vi "Main.vi"() -> ()   [LabVIEW 2015]
uses:
  Ctrls/btnCloseWin.ctl
  Ctrls/YesOrNo.ctl
  Ctrls/btnAboutNew.ctl
  Ctrls/btnDonateNew.ctl
  Ctrls/btnMinSizeWin.ctl
  Ctrls/btnMaxSizeWin.ctl
  Ctrls/btnUpdateNew.ctl
  Ctrls/btnOpenDBplusplus.ctl
  Ctrls/btnOpenCANtest.ctl
  Ctrls/btnOpenCANpro.ctl
  Ctrls/btnOpenZCANPRO.ctl
  Ctrls/btnSetupNew.ctl
  Ctrls/SettingParameters.ctl
  Ctrls/btnOpenDBC.ctl
  Ctrls/btnOpenData.ctl
  Ctrls/btnOpenTSmaster.ctl
  Ctrls/btnOpenOrigin.ctl
  <vilib>/Utility/sysdir.llb/System Directory Type.ctl
  <vilib>/Platform/TimedLoop/XDataNode/timing_clust.ctl
  <vilib>/Platform/TimedLoop/XDataNode/nitl_modes.ctl
  <vilib>/Platform/TimedLoop/XDataNode/wakeup.ctl
  <vilib>/Utility/miscctls.llb/LVPointTypeDef.ctl
  <vilib>/Utility/miscctls.llb/LVRectTypeDef.ctl
  SubVIs/GlobalVar.vi
  GlobalVariables.vi
  <vilib>/Utility/config.llb/Write Key (Boolean).vi
  <vilib>/Utility/config.llb/Read Key (Path).vi
  <vilib>/Utility/config.llb/Write Key (Path).vi
  <vilib>/Utility/config.llb/Read Key (Boolean).vi
  <vilib>/Utility/NIReport.llb/Append Text Table to Report (wrap).vi
  <vilib>/Platform/TimedLoop/XDataNode/XDataNode.xnode
  <vilib>/Utility/NIReport.llb/NI_report.lvclass
  <vilib>/Utility/config.llb/NI_LVConfig.lvlib
  <vilib>/Platform/TimedLoop/XDataNode/XDNodeRunTimeDep.lvlib
  <vilib>/Utility/NIReport.llb/Excel/NI_Excel.lvclass
panel:
  out "CursorNum2":dbl
  out "CursorNum1":dbl
  out "CursorTXT2":string
  out "CursorTXT1":string
  out "MainGrapgDraw_finished":bool
  out "Data_loaded":bool
  out "DBC_loaded":bool
  in  "btnMultiDecAndExp":bool caption="boolExport2Excel"
  in  "btnOpenOrigin":T1
  in  "btnOpenTSmaster":T2 caption="btnOpenCANpro"
  out "Y_DisplayNum":i32
  in  "ZoomMode":u16(ring) items=["Zoom：XY", "Zoom：X", "Zoom：Y1", "Zoom：Y2", "Zoom：Y3", "Zoom：Y4", "Zoom：Y5", "Zoom：Y6", "Zoom：Y7", "Zoom：Y8", "Zoom: All Y"]
  out "MporofSelSgs":string[][](array[string]) caption="已选信号数组"
  in  "btnOpenCANData":T3
  out "CANDatafileIn":string caption="CAN离线数据（.can/.txt/.csv/.asc/.trc/.blf）"
  in  "btnOpenDBC":T4
  out "DBCfileIn":string caption="DBC文件(.dbc)"
  in  "dbcSigOver1":bool
  in  "isShowYValue":T5=TRUE caption="AutoLine"
  in  "isShowXY":T5=TRUE caption="AutoLine"
  out "SelectedSigValListArry":string[][](array[string]) caption="值表数组"
  in  "LineWidth":u8
  out "XYTips":string
  out "ChkUpdateCnt":i32
  out "ReadSettingsReady":bool=TRUE
  out "Settings":T6 {"ChkUpdatePeriod" items=["EveryMonth"=2592000, "EveryWeek"=604800, "Everyday"=86400, "EveryHour"=3600, "EveryLaunch"=1, "Never"=0]}
  in  "btnConfigYandCurves":bool caption="配置纵坐标"
  in  "isAutoCurves":T5=TRUE caption="AutoLine"
  in  "isAutoY":T5=TRUE caption="AutoY"
  in  "TimeFormat":u16(ring) items=["Relative(s)", "Abs(noDate)", "Abs(withDate)"]
  in  "isTimeRerange":T5=TRUE caption="AutoY"
  out "Language":u32
  in  "btnSetup":T7
  in  "btnOpenZCANPRO":T8
  in  "btnOpenCANpro":T9
  in  "btnOpenCANtest":T10
  in  "btnOpenDBplus2":T11
  in  "btnUpdateChk":T12
  in  "btnMax":T13
  in  "btnMin":T14
  in  "btnCANFileInfo":bool caption="空白按钮"
  out "CANMessagesAllInfo":string[][](array[string])
  out "XYGraphData":cluster{"时间(s)":dbl[], "数据":dbl[]}[](array[cluster])
  out "BaseTimeCluster":T15
  in  "boolMergeFiles":bool caption="空白按钮"
  in  "btnDonate":T16
  in  "btnAbout":T17
  in  "ClusterSigFormat":T18
  out "CurveCustomSealedArray":string[][](array[string]) caption="已选信号数组"
  out "CanMessageRowsNum":i32 caption="帧数"
  out "FileSize":dbl caption="文件大小" format="%.2f MB"
  out "ManuCofigofYaxle":cluster{"Y轴序号":u8, "Y轴名称":string, "可见性":bool}[](array[cluster])
  out "ManuCofigofCurves":T19(array[cluster])
  in  "boolExport2Excel":bool
  out "LastCANPath":path
  out "LastDBCPath":path
  out "isDataLoaded":bool caption="离线数据已加载"
  out "DataArryOfCANLoaded":u32[][](array[numeric]) caption="加载的CAN离线数据数组"
  out "ProgressNumerical":string="0%" caption="进度数值"
  out "HorizontalProgressBar":u8(slide) caption="水平进度条" scale=0.0..100.0
  out "SigValListArry":string[][](array[string]) caption="值表数组"
  in  "LookAllSigDefinition":bool caption="查看所有值表"
  in  "LookSelSigDefinition":bool caption="查看已选值表"
  in  "AllValueTable":string(tree) caption="所有ValueTable"
  out "txtDrawingPrompt":string="让我看看有多少数据..." caption="绘图提示语"
  in  "GraphLegendWidth":u32 caption="图例与游标宽度"
  in  "ClearMainGraph":bool caption="清空主图"
  out "NumSelected":i32 caption="已选数量"
  in  "ListOfDBC":string(tree) caption="DBC一览树形"
  in  "boolLoadLastDBC":bool caption="空白按钮"
  in  "ClearSelectedSig":bool caption="清空选择"
  out "CANmessageNum":i32 caption="报文数"
  out "SigNum":i32 caption="信号数"
  in  "DBCpath":path caption="DBC文件（.dbc）"
  in  "CANpath":path caption="CAN离线数据（.can/.txt/.csv/.asc/.trc）"
  out "ArrySelectedSig":string[][](array[string]) caption="已选信号数组"
  out "DBCAllSigArry":string[][](array[string]) caption="全部信号数组"
  in  "boolDrawGraph":bool caption="绘图"
  in  "btnExit":T20 caption="退出"
  in  "SelectedSigList":i32(listbox)=-1 caption="已选信号列表"
  out "MainGraph":cluster{"时间(s)":dbl[], "数据":dbl[]}[](graph) caption="时域主图"
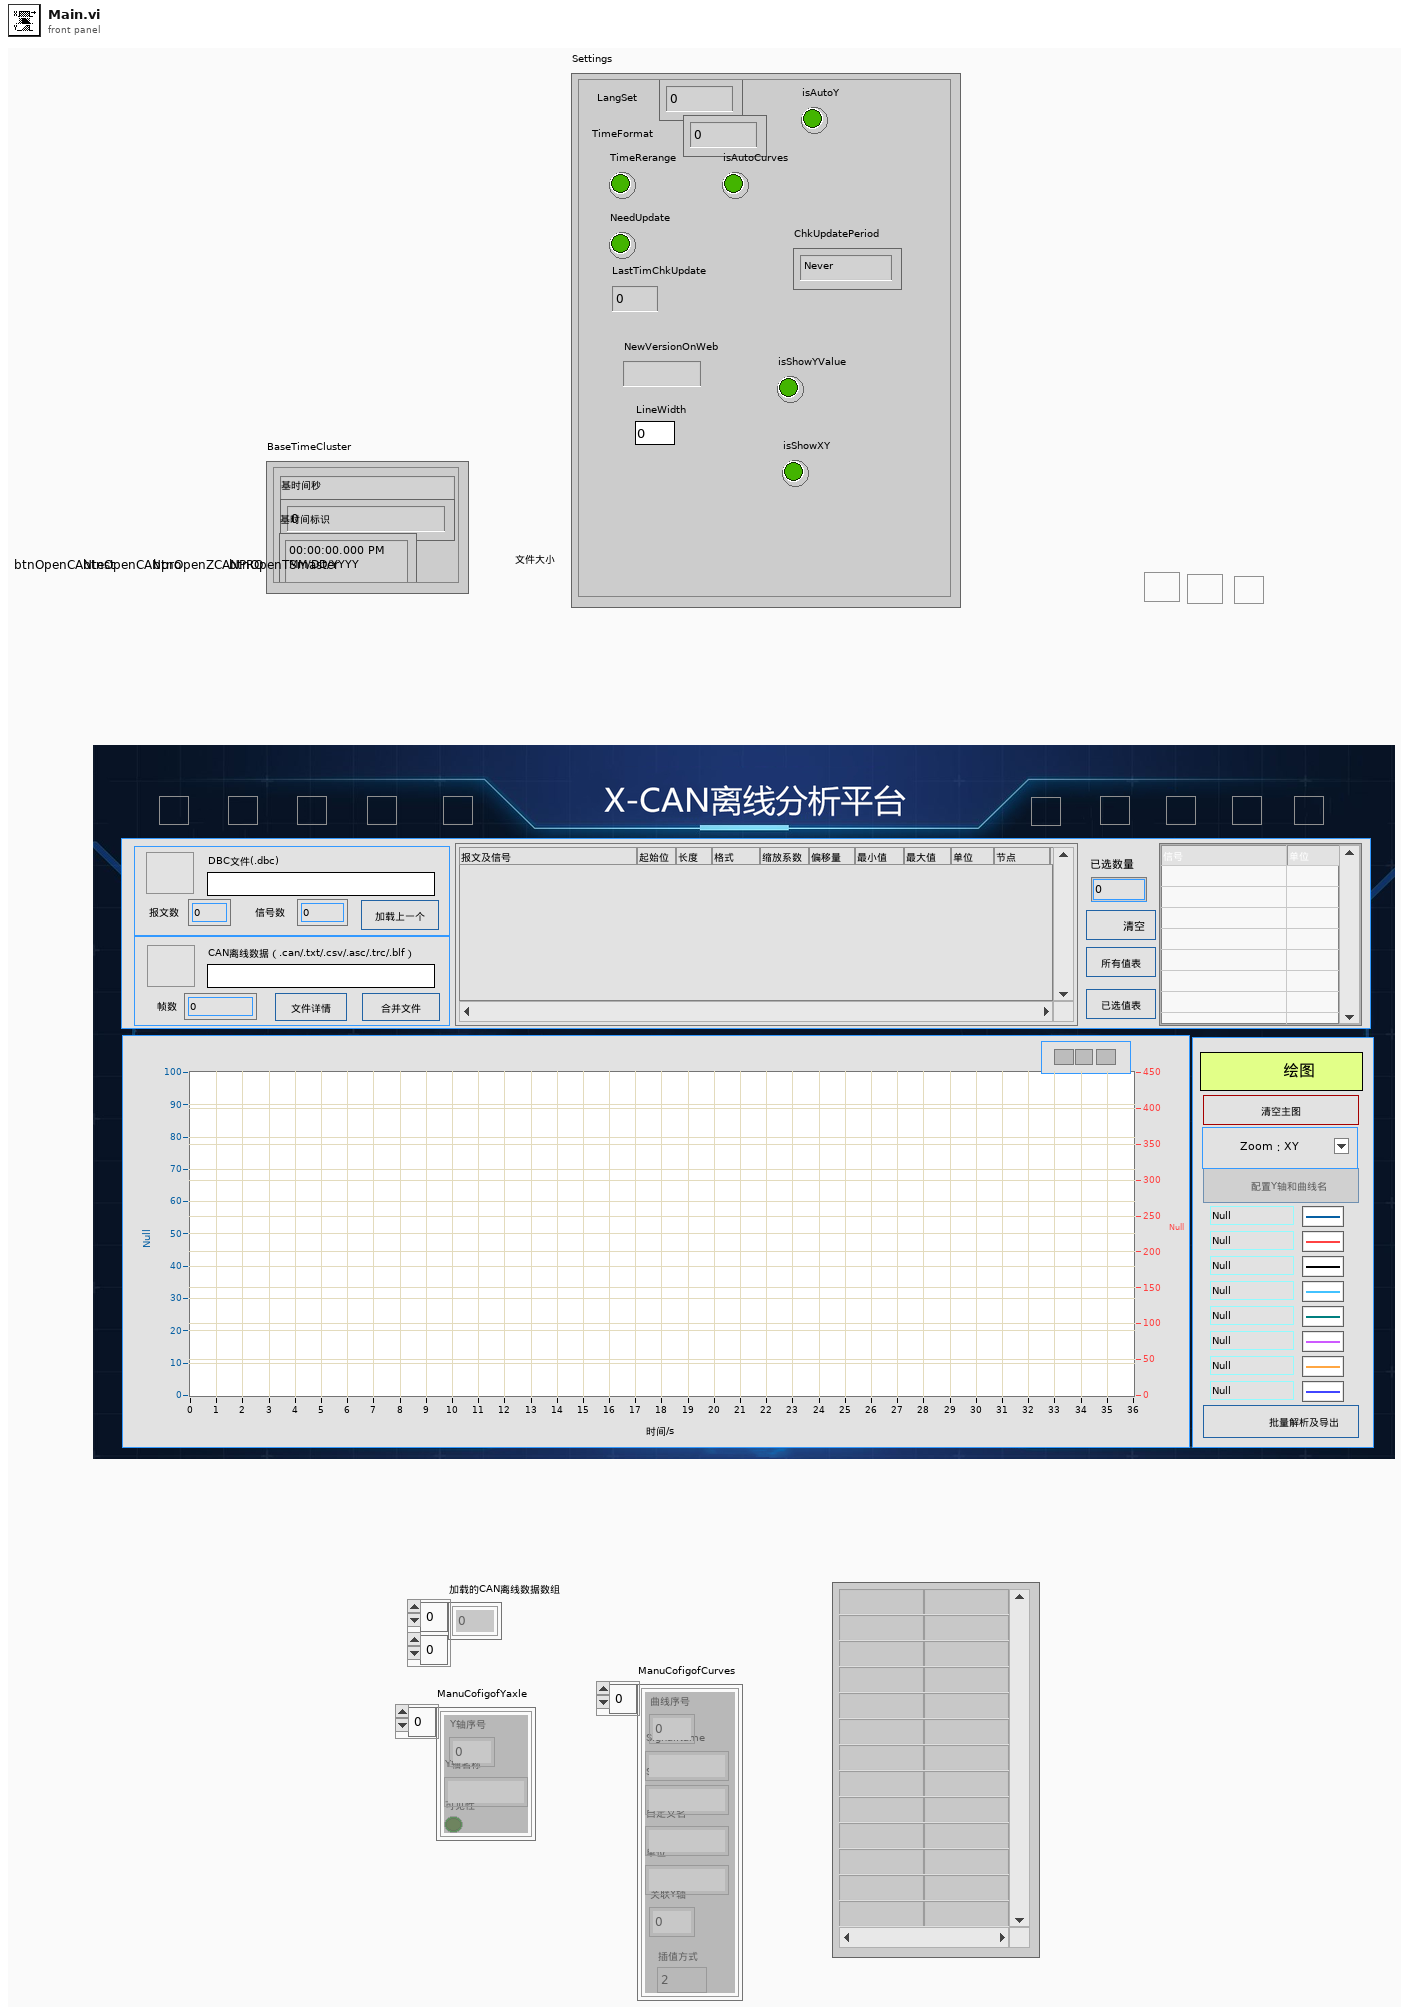
[diagram p1: front panel]
types:
  T1 = typedef "btnOpenOrigin.ctl" = bool
  T2 = typedef "btnOpenTSmaster.ctl" = bool
  T3 = typedef "btnOpenData.ctl" = bool
  T4 = typedef "btnOpenDBC.ctl" = bool
  T5 = typedef "YesOrNo.ctl" = bool
  T6 = typedef "SettingParameters.ctl" = cluster{"LangSet":u32, "TimeFormat":u16, "TimeRerange":bool, "isAutoCurves":bool, "isAutoY":bool, "NeedUpdate":bool, "LastTimChkUpdate":dbl, "NewVersionOnWeb":string, "ChkUpdatePeriod":u32, "LineWidth":u8, "isShowYValue":bool, "isShowXY":bool}
  T7 = typedef "btnSetupNew.ctl" = bool
  T8 = typedef "btnOpenZCANPRO.ctl" = bool
  T9 = typedef "btnOpenCANpro.ctl" = bool
  T10 = typedef "btnOpenCANtest.ctl" = bool
  T11 = typedef "btnOpenDBplusplus.ctl" = bool
  T12 = typedef "btnUpdateNew.ctl" = bool
  T13 = typedef "btnMaxSizeWin.ctl" = bool
  T14 = typedef "btnMinSizeWin.ctl" = bool
  T15 = cluster{"基时间字符串":string, "基时间秒":dbl, "基时间标识":timestamp}
  T16 = typedef "btnDonateNew.ctl" = bool
  T17 = typedef "btnAboutNew.ctl" = bool
  T18 = cluster{"起始位":u8, "长度":u8, "缩放系数":dbl, "偏移量":dbl, "符号":string}
  T19 = cluster{"曲线序号":u8, "SignalName":string, "SignalTag":string, "自定义名":string, "单位":string, "关联Y轴":u8, "插值方式":dbl}[]
  T20 = typedef "btnCloseWin.ctl" = bool
  T21 = typedef "System Directory Type.ctl" = i32
  T22 = typedef "XDNodeRunTimeDep.lvlib/timing_clust.ctl" = cluster{"Expected End [f-1]":u64, "Actual End [f-1]":u64, "Finished Late? [f-1]":bool, "Expected End [i-1]":u64, "Actual End [i-1]":u64, "Finished Late? [i-1]":bool, "Expected Start [i]":u64, "Actual Start [i]":u64, "Expected Start [f]":u64, "Actual Start [f]":u64, "Source Name":string, "Structure Name":string, "Period":i64, "Deadline":i64, "Offset":i64, "Start":i64, "Priority":i32, "Timeout":i32, "Mode":T23, "Wakeup Reason":T24, "Error":errorcluster, "Source Type":string, "Secondary Source Type":string, "Global End Time":u64, "Global Start Time":u64, "Frame Duration":u64, "Iteration Duration":u64, "Assigned CPU":i32, "I/O Scan Engine Mode":u32}
  T23 = typedef "XDNodeRunTimeDep.lvlib/nitl_modes.ctl" = enum32{"No Change", "Process missed periods, maintain original phase", "Discard missed periods, maintain original phase", "Process missed periods, ignore original phase", "Discard missed periods, ignore original phase"}
  T24 = typedef "XDNodeRunTimeDep.lvlib/wakeup.ctl" = enum32{"Normal", "Aborted", "Asynchronous wakeup", "Timing source error", "Timed loop error", "Timeout"}
  T25 = typedef "LVPointTypeDef.ctl" = cluster{"Horizontal":i16, "Vertical":i16}
  T26 = typedef "LVRectTypeDef.ctl" = cluster{"Left":i16, "Top":i16, "Right":i16, "Bottom":i16}
  T27 = enum8{"Enabled", "Disabled", "Disabled and Grayed Out"}
  T28 = enum32{"Invalid", "Standard", "Closed", "Hidden", "Minimized", "Maximized"}
  T29 = cluster{"left":i32, "top":i32, "right":i32, "bottom":i32}
  T30 = typedef "NI_LVConfig.lvlib/Config Data RefNum.ctl" = refnum<k1>
  T31 = cluster{"Visible":bool, "Color":u32, "LineWidth":u8}
  T32 = typedef "LVPoint32TypeDef.ctl" = cluster{"Horizontal":i32, "Vertical":i32}
  T33 = typedef "LVRowAndColumnTypeDef.ctl" = cluster{"Row":i32, "Column":i32}
  T34 = typedef "配置Y轴按钮.ctl" = bool
  T35 = cluster{"Shift":bool, "Ctrl":bool, "Alt":bool, "Cmd":bool, "Opt":bool}
  T36 = cluster{"Ylimits":cluster{"Upbound":dbl, "Downbound":dbl}, "ParentScaleID":i32, "LabelTitle":string}
  T37 = typedef "LVPointDoubleTypeDef.ctl" = cluster{"Cursor X":dbl, "Cursor Y":dbl}
  T38 = enum16{"maximized", "minimized", "normal", "no change"}
  T39 = enum16{"Standard Report", "HTML", "Word", "Excel"}
  T40 = cluster{"Color":u32, "PointStyle":u8, "LineStyle":u8, "Interp":u8, "LineWidth":u8, "BarPlotStyle":u8, "FillTo":i16, "XScaleIdx":u32, "YScaleIdx":u32, "Anti-Aliased":bool, "LabelFormat":u8, "TransitionType":u8, "TransitionLocation":u8, "DigitalLineStyle":u8}
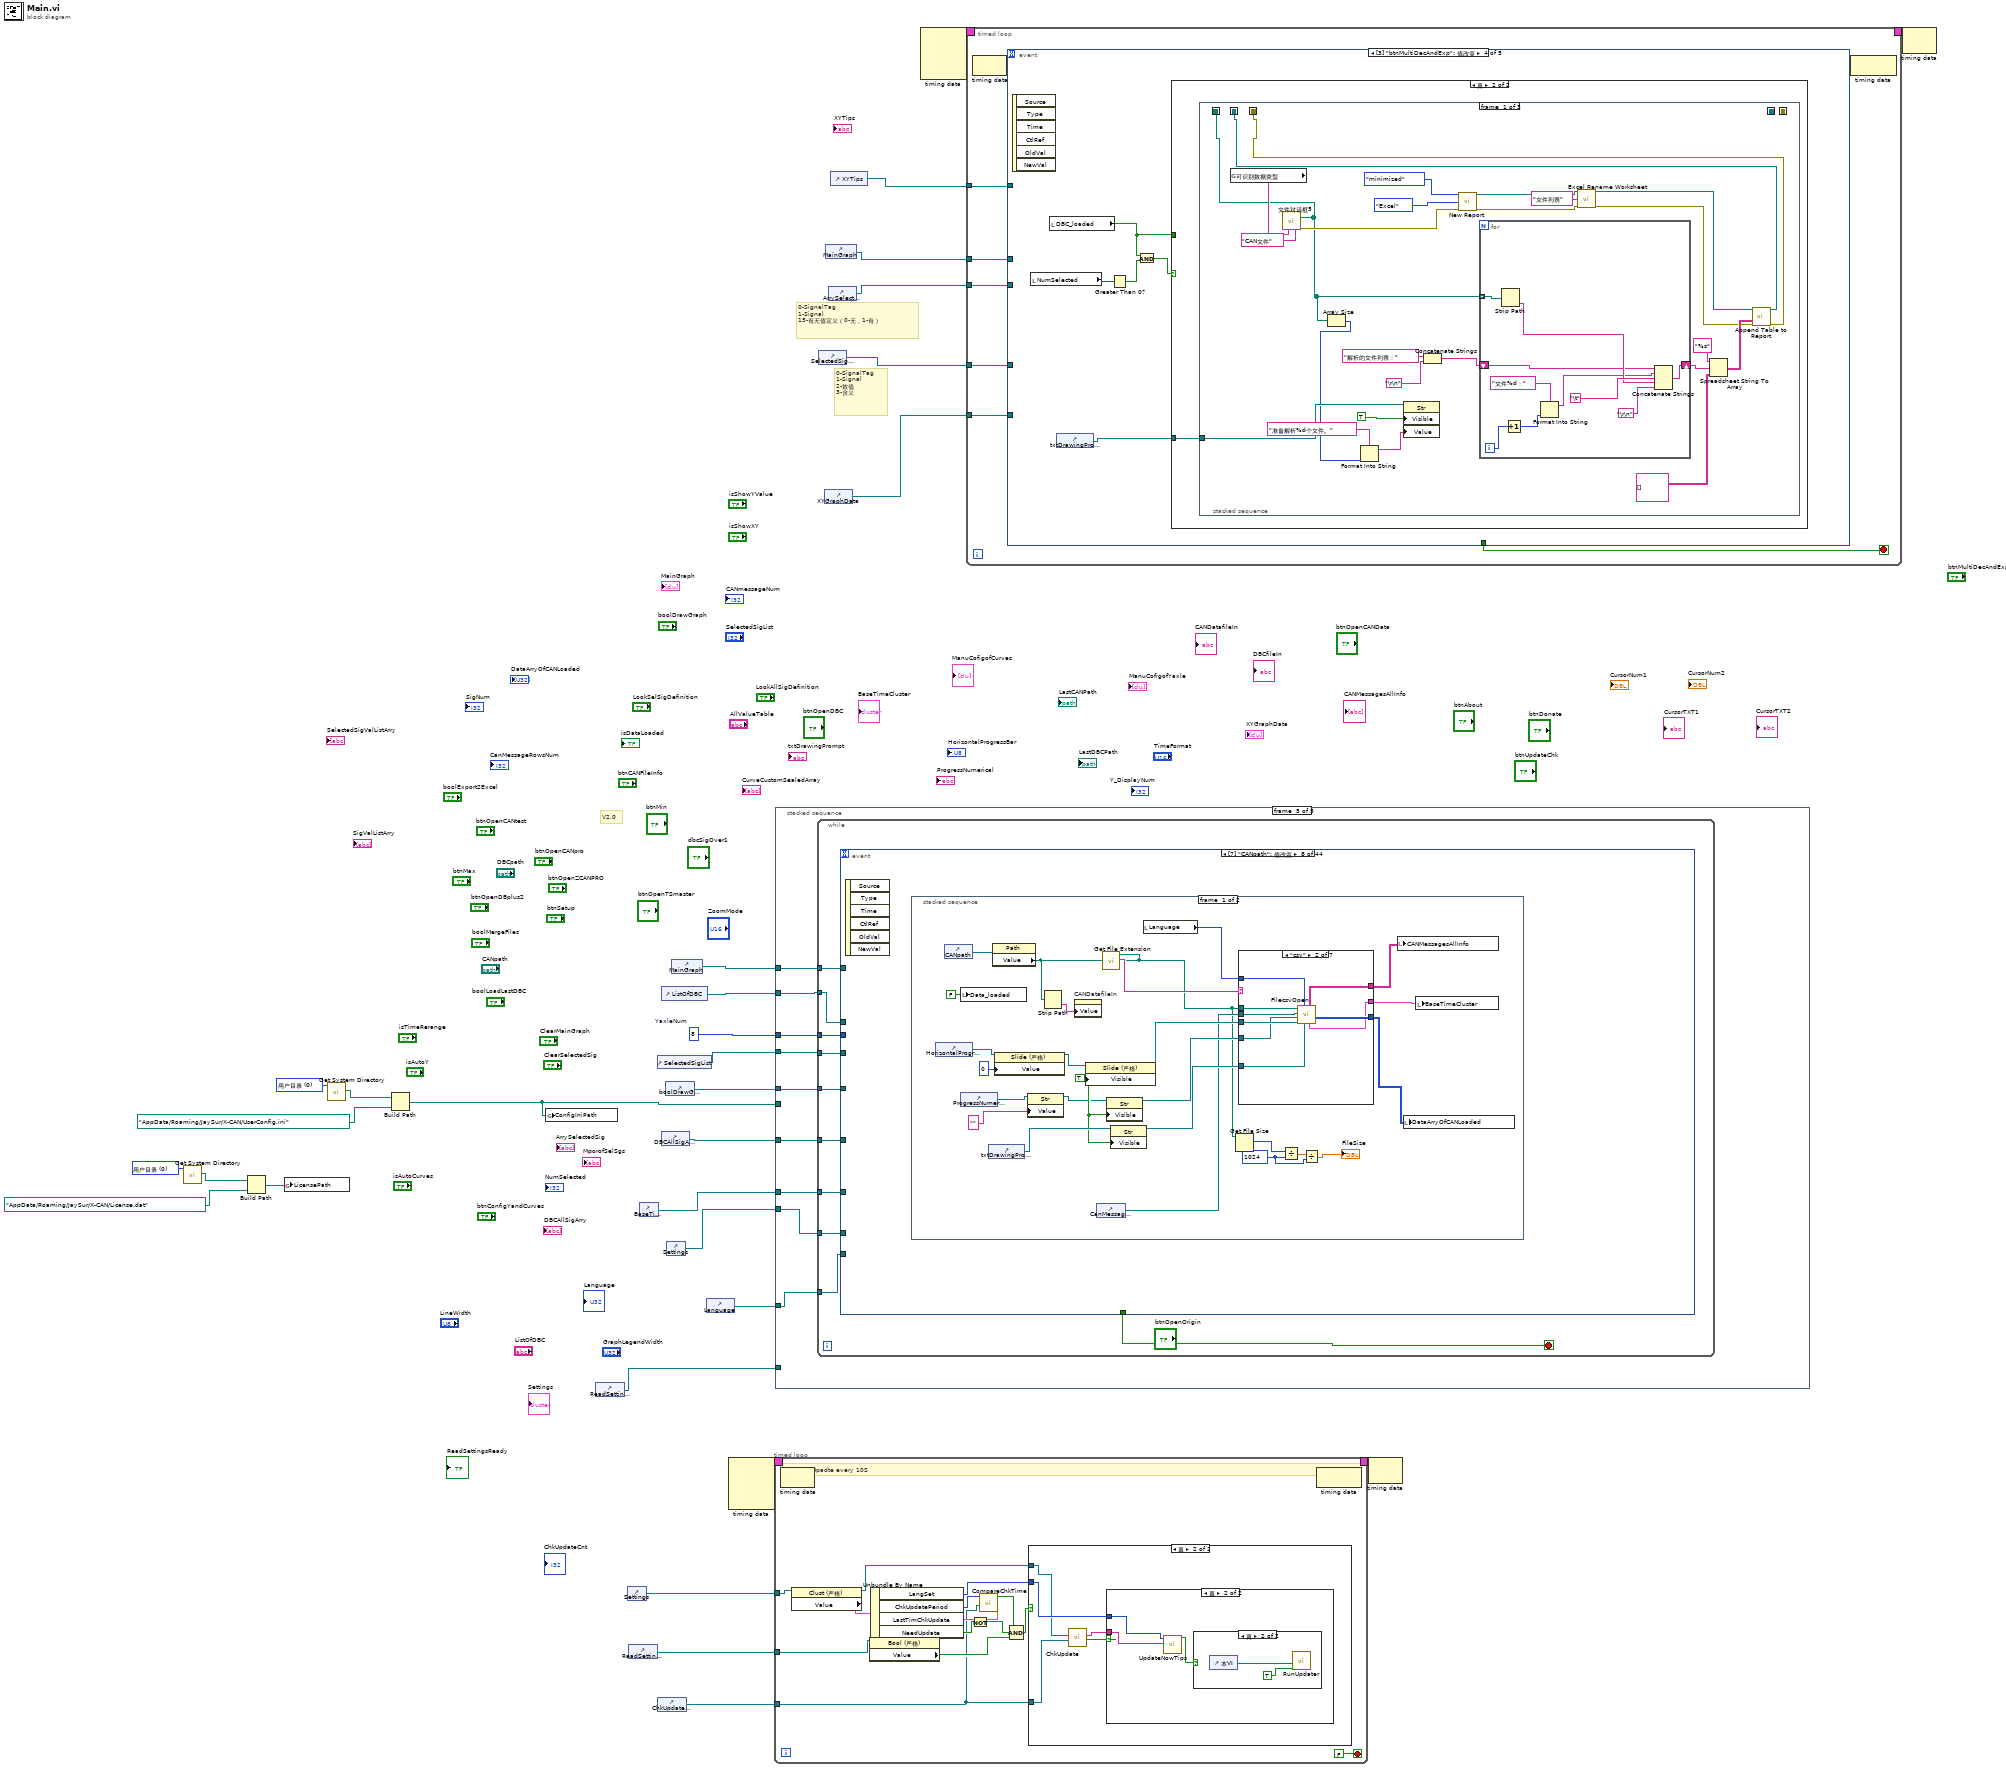
[diagram p0: block diagram]
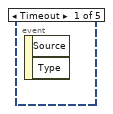
[diagram p2: hidden frame]
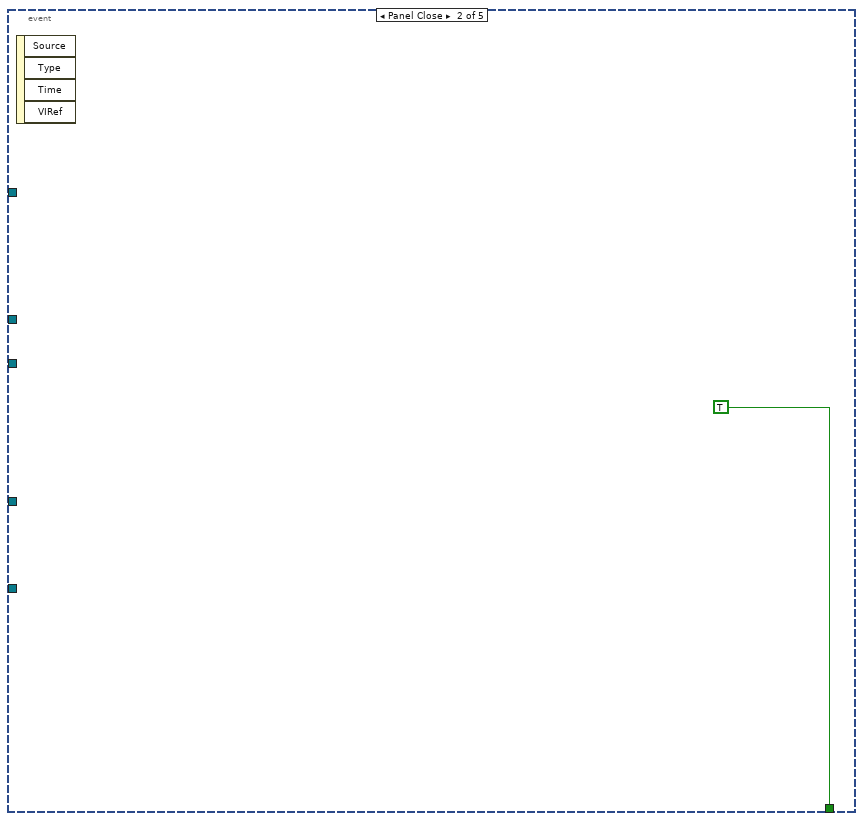
[diagram p3: hidden frame]
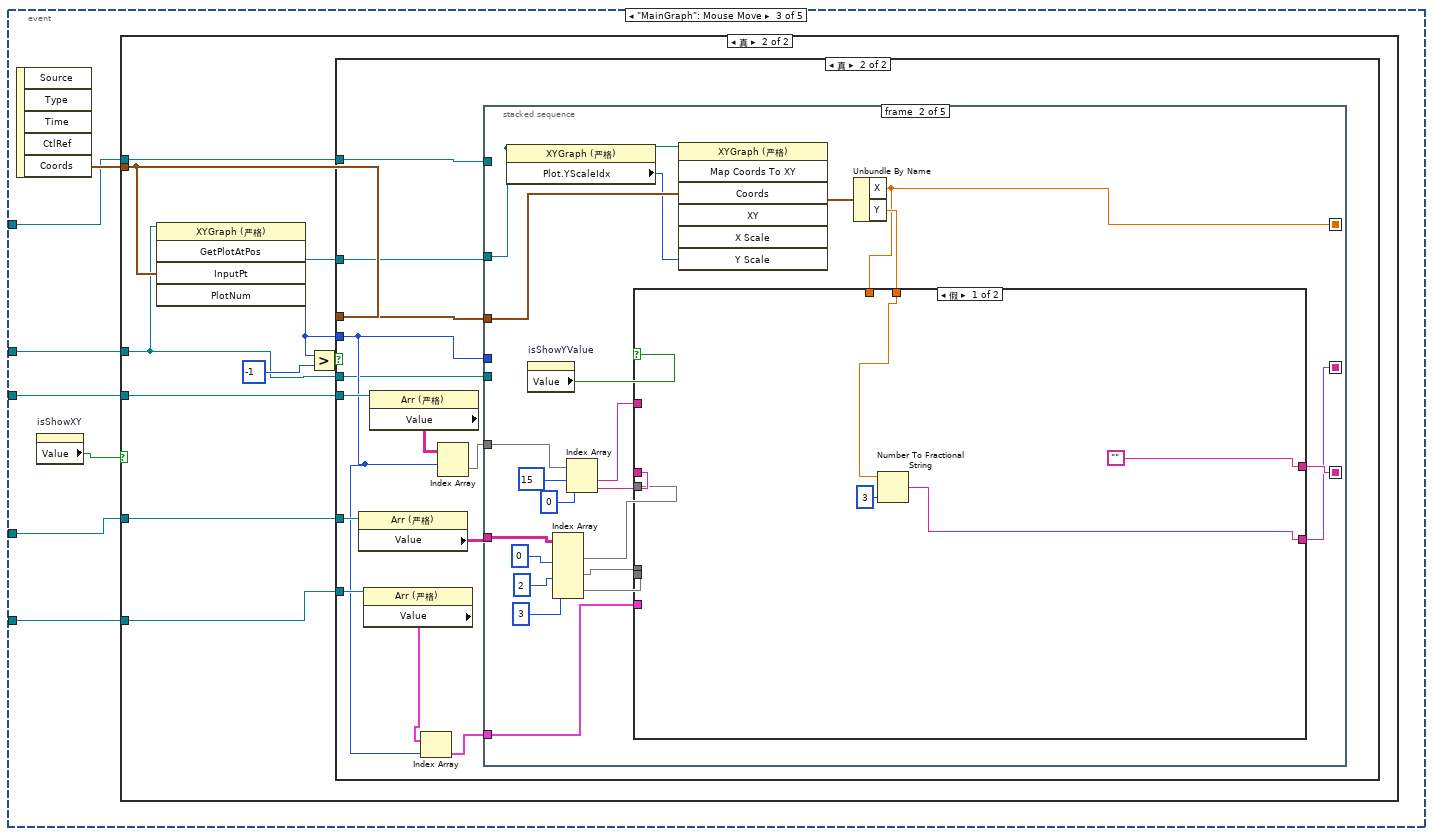
[diagram p4: hidden frame]
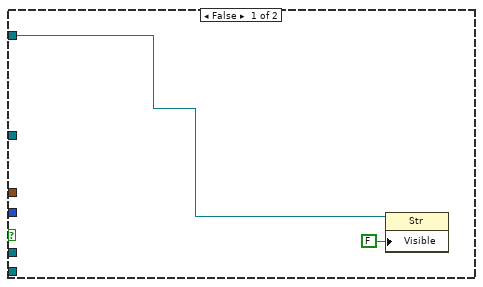
[diagram p6: hidden frame]
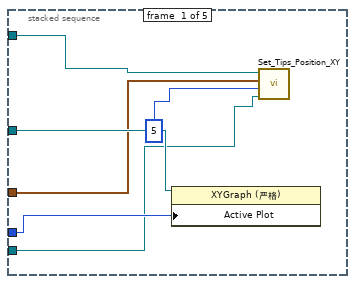
[diagram p7: hidden frame]
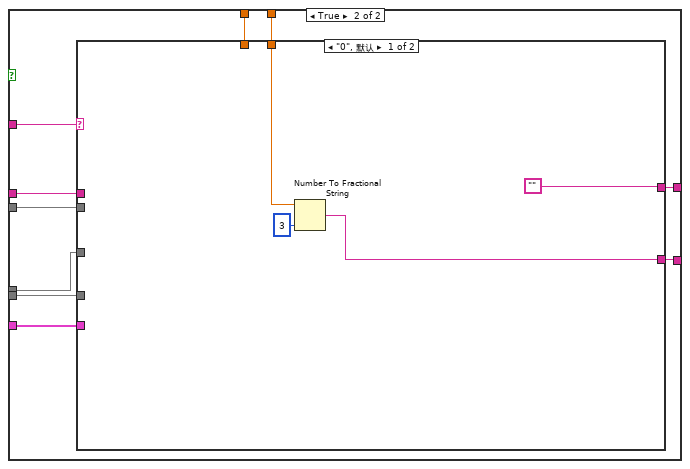
[diagram p8: hidden frame]
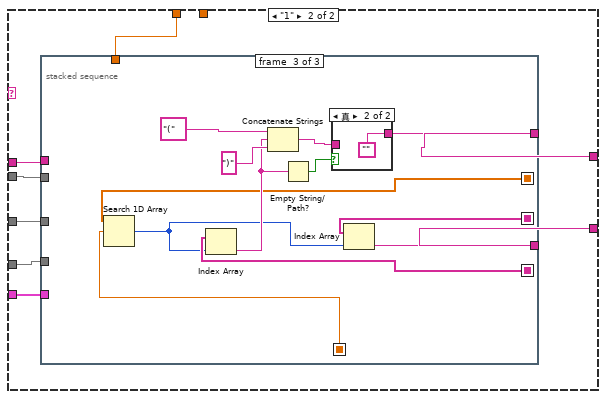
[diagram p9: hidden frame]
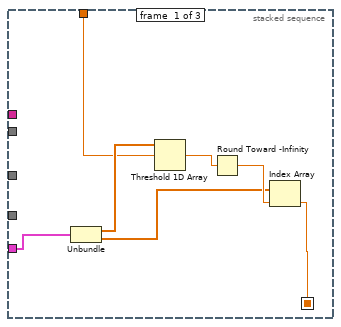
[diagram p10: hidden frame]
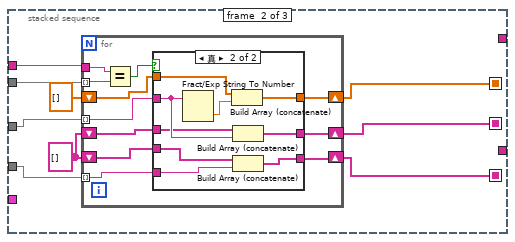
[diagram p11: hidden frame]
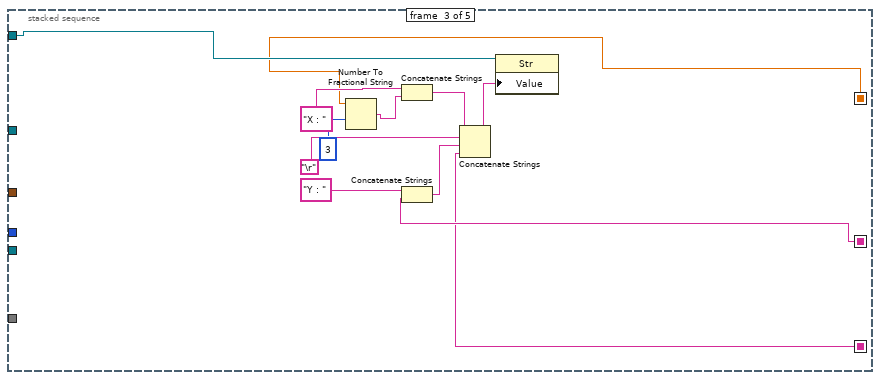
[diagram p14: hidden frame]
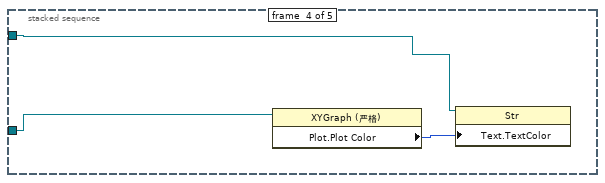
[diagram p15: hidden frame]
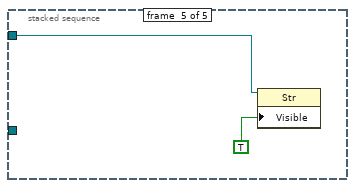
[diagram p16: hidden frame]
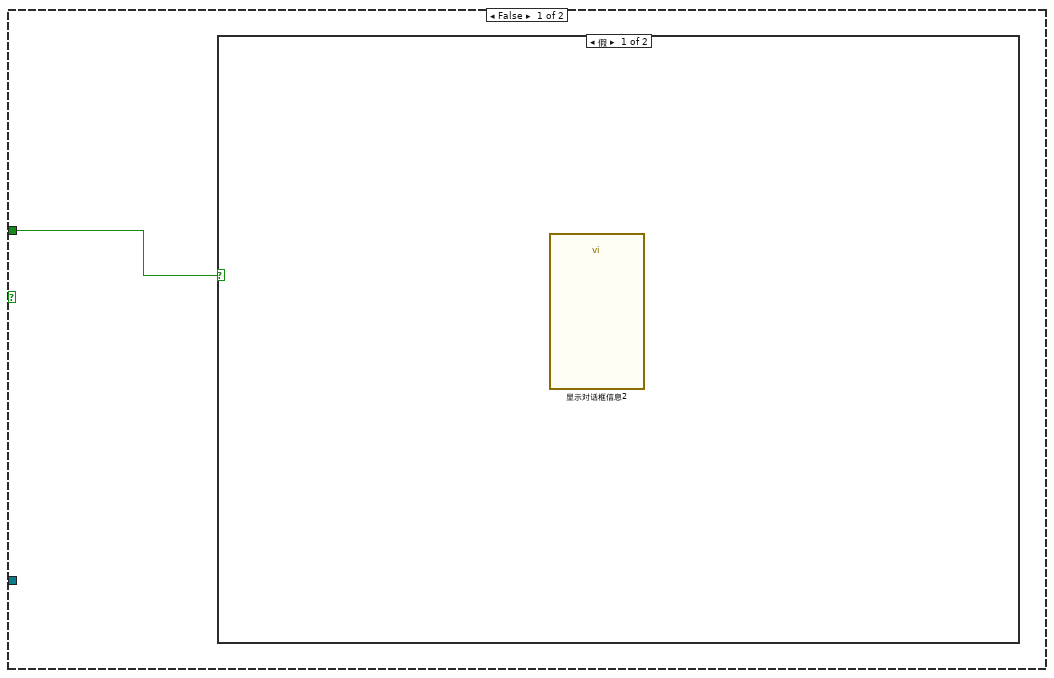
[diagram p17: hidden frame]
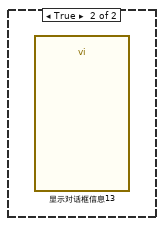
[diagram p18: hidden frame]
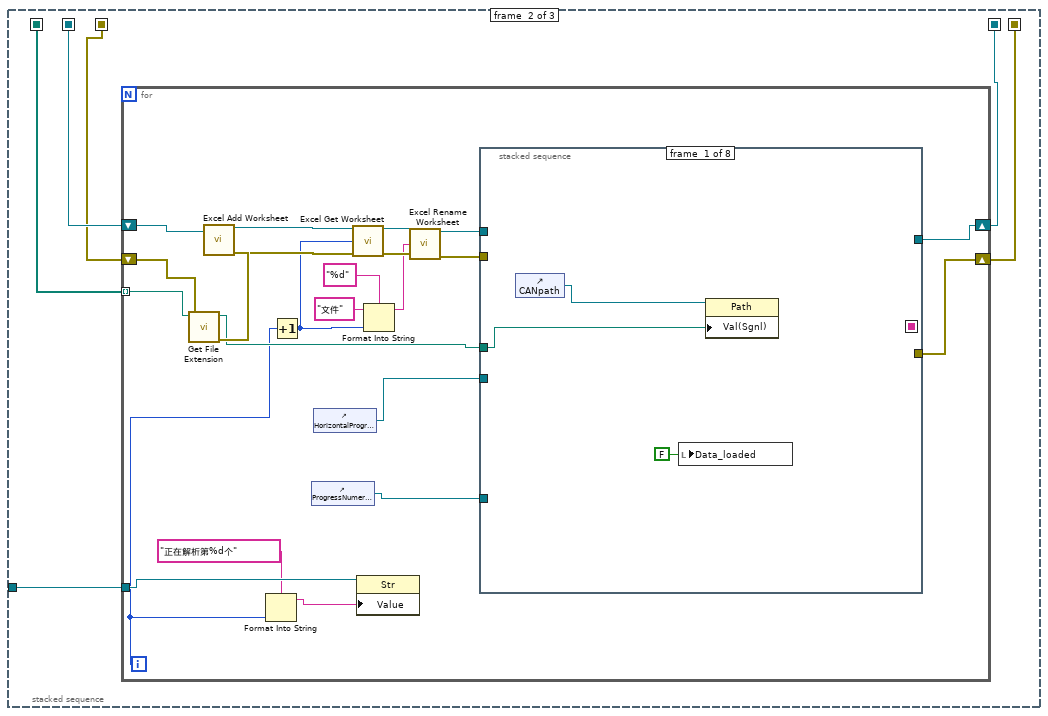
[diagram p19: hidden frame]
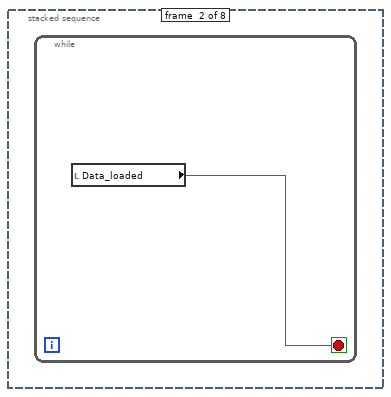
[diagram p20: hidden frame]
diagram:
  w4 = T21 0 items=["用户目录"=0, "用户桌面"=1, "用户文档"=2, "用户应用程序数据"=3, "用户设置"=4, "用户临时目录"=5, "公共文档"=6, "公共应用程序数据"=7, "公共设置"=8, "公共缓存"=13, "系统核心库"=9, "系统安装库"=10, "应用程序文件"=11, "启动盘根目录"=12] ("system directory type")
  w23 = T21 0 items=["用户目录"=0, "用户桌面"=1, "用户文档"=2, "用户应用程序数据"=3, "用户设置"=4, "用户临时目录"=5, "公共文档"=6, "公共应用程序数据"=7, "公共设置"=8, "公共缓存"=13, "系统核心库"=9, "系统安装库"=10, "应用程序文件"=11, "启动盘根目录"=12] ("system directory type")
  w30 = 8  # YaxleNum
  # "0-SignalTag\n1-Signal\n2-数值\n3-含义"
  # "0-SignalTag\n1-Signal\n15-有无值定义（0-无，1-有）"
  # "V2.0"
  n1 = call <vilib>:"Get System Directory.vi"("system directory type"=w4) -> ("system directory"=w3:path)  [unwired: 10 in]
  n2 = Build Path(base path=w3, name or relative path=path "AppData/Roaming/JaySur/X-CAN/License.dat" ("default name")) -> (appended path=w2:path)
  n3 = global write "GlobalVar.vi" "LicensePath"(w2) -> ()
  n4 = call <vilib>:"Get System Directory.vi"("system directory type"=w23) -> ("system directory"=w22:path)  [unwired: 10 in]
  n5 = Build Path(base path=w22, name or relative path=path "AppData/Roaming/JaySur/X-CAN/UserConfig.ini" ("default name")) -> (appended path=w1:path)
  n6 = global write "GlobalVar.vi" "ConfigIniPath"(w1) -> ()
  n7 = control-ref of="ReadSettingsReady"() -> (w18:refnum<vi>)
  n8 = control-ref of="Settings"() -> (w19:refnum<vi>)
  n9 = control-ref of="ReadSettingsReady"() -> (w17:refnum<vi>)
  n10 = control-ref of="BaseTimeCluster"() -> (w24:refnum<vi>)
  n11 = control-ref of="SelectedSigList"() -> (w27:refnum<vi>)
  n12 = control-ref of="ChkUpdateCnt"() -> (w15:refnum<vi>)
  n13 = control-ref of="ListOfDBC"() -> (w28:refnum<vi>)
  n14 = control-ref of="DBCAllSigArry"() -> (w29:refnum<vi>)
  n15 = control-ref of="boolDrawGraph"() -> (w11:refnum<vi>)
  n16 = control-ref of="Settings"() -> (w16:refnum<vi>)
  n17 = control-ref of="MainGraph"() -> (w26:refnum<vi>)
  n18 = control-ref of="Language"() -> (w6:refnum<vi>)
  n19 = node-c288() -> (w21:T22)  [unwired: 4 in]
  n20 = timed-loop {
    timing: w21 -> [_]
    timing-out: [_] -> w20
    tunnel: w19 -> [w31]
    tunnel: w17 -> [w40]
    tunnel: w15 -> [w33]
    stop <- FALSE stop-if-true
    # "Checking Upadte every 10S"
    n21 = node-c288() -> ()  [unwired: 1 in, 1 out]
    n22 = property class="Clust (严格)"(reference=w31) -> (reference out=w41:refnum<vi>, "Value"=w44:T6)  [unwired: 1 in, 1 out]
    n23 = property class="Bool (严格)"(reference=w40) -> ("Value"=w39:bool)  [unwired: 1 in, 2 out]
    n24 = Unbundle By Name(w44) -> ("LangSet"=w34:u32, "ChkUpdatePeriod"=w35:u32, "LastTimChkUpdate"=w43:dbl, "NeedUpdate"=w42:bool)
    n25 = Not(x=w42) -> (.not. x?=w38:bool)
    n26 = call "CompareChkTime.vi"("ChkUpdateCnt"=w33, "LastTimChkUpdate"=w43, "ChkUpdatePeriod"=w35) -> ("OK2Chk"=w37:bool)  [unwired: 8 in]
    n27 = Compound Arithmetic op=AND ("复合运算")(w37, w38, w39) -> (w36:bool)
    n28 = case shown="真" w36 {
      tunnel: w41 -> [_ w45]
      tunnel: w34 -> [_ w48]
      tunnel: w33 -> [_ w47]
      frame False {
      }
      frame True {
        n29 = call "ChkUpdate.vi"("ChkUpdateCnt"=w47, "Settings"=w45) -> ("FoundNew"=w49:bool, "NewVersion"=w46:string)  [unwired: 8 in]
        n30 = case shown="真" w49 {
          tunnel: w48 -> [_ w51]
          tunnel: w46 -> [_ w50]
          frame False {
          }
          frame True {
            n31 = call "UpdateNowTips.vi"("NewVersionOnWeb"=w50, "LangSet"=w51) -> ("UpdateNow"=w52:bool)  [unwired: 9 in]
            n32 = case shown="真" w52 {
              frame False {
              }
              frame True {
                n33 = control-ref of="本VI"() -> (w53:refnum<vi>)
                n34 = call "RunUpdater.vi"("关闭前面板"=TRUE, "VI输入"=w53) -> ()  [unwired: 10 in]
              }
            }
          }
        }
      }
    }
    n35 = node-c288() -> ()  [unwired: 1 in, 1 out]
  }
  n36 = stacked-sequence {
    tunnel: w30 -> [_ _ w250 _ w280]
    tunnel: w29 -> [_ _ _ _ w279]
    tunnel: w28 -> [_ w182 _ _ w278]
    tunnel: w26 -> [_ w180 w231 w267 w277]
    tunnel: w27 -> [_ _ _ w269 w276]
    tunnel: w1 -> [_ w161 _ _ _]
    tunnel: w24 -> [_ _ _ _ w275]
    tunnel: w18 -> [_ w168 w238 _ _]
    tunnel: w16 -> [_ w165 _ _ w274]
    tunnel: w11 -> [_ _ _ _ w273]
    tunnel: w6 -> [_ _ _ _ w272]
    frame #0 {
      n37 = control-ref of="本VI"() -> (w73:refnum<vi>)
      n38 = call "LV_GetSysMetrics.vi"() -> ("UserMetrics"=w66:cluster{"UserWidth":i32, "UserHeight":i32}, "Rect"=w62:T29, "SM_CYSIZE"=w64:i32)  [unwired: 8 in, 1 out]
      n39 = property class="VI"(reference=w73) -> (reference out=w72:refnum<vi>, "Minimum Panel Size"=w60:T25)  [unwired: 1 in, 1 out]
      n40 = Unbundle By Name(w66) -> ("UserWidth"=w71:i32, "UserHeight"=w70:i32)
      n41 = Add(x=T25 {"Horizontal"=5, "Vertical"=5}, y=w60) -> (x+y=w58:T25)
      n42 = Unbundle By Name(w58) -> ("Horizontal"=w61:i16, "Vertical"=w65:i16)
      n43 = Add(x=w64, y=w65) -> (x+y=w63:i32)
      n44 = Less Or Equal?(x=w71, y=w61) -> (x <= y?=w68:bool)
      n45 = Less Or Equal?(x=w70, y=w63) -> (x <= y?=w69:bool)
      n46 = Or(x=w68, y=w69) -> (x .or. y?=w67:bool)
      n47 = case shown="假" w67 {
        tunnel: w66 -> [w86 w117]
        tunnel: w72 -> [w84 w107]
        tunnel: w60 -> [_ _]
        tunnel: w64 -> [_ _]
        tunnel: w63 -> [w78 w111]
        tunnel: w62 -> [_ w118]
        tunnel: w61 -> [_ w115]
        tunnel: w58 -> [w75 _]
        frame False {
          n48 = Unbundle By Name(w86) -> ("UserWidth"=w97:i32)
          n49 = Unbundle By Name(w75) -> ("Horizontal"=w77:i16)
          n50 = Unbundle By Name(w86) -> ("UserHeight"=w85:i32)
          n51 = Subtract(x=w97, y=w77) -> (x-y=w96:i32)
          n52 = Subtract(x=w85, y=w78) -> (x-y=w87:i32)
          n53 = Divide(x=w96, y=2) -> (x/y=w93:dbl)
          n54 = Divide(x=w87, y=2) -> (x/y=w90:dbl)
          n55 = Greater Or Equal To 0?(x=w93) -> (x >= 0?=w94:bool)
          n56 = Greater Or Equal To 0?(x=w90) -> (x >= 0?=w89:bool)
          n57 = Select(t=w93, s=w94, f=0 ("y")) -> (s? t:f=w83:dbl)
          n58 = Select(t=w90, s=w89, f=0 ("y")) -> (s? t:f=w81:dbl)
          n59 = Add(x=w83, y=w77) -> (x+y=w82:dbl)
          n60 = Add(x=w81, y=w78) -> (x+y=w80:dbl)
          n61 = Bundle By Name(cluster=T26 {"Left"=0, "Top"=0, "Right"=0, "Bottom"=0} ("输出簇"), "Left"=w83, "Top"=w81, "Right"=w82, "Bottom"=w80) -> (w79:T26)
          n62 = property class="VI"(reference=w84, "Front Panel.WinBounds"=w79) -> (error out=w74:errorcluster)  [unwired: 1 in, 1 out]
          n63 = call <vilib>:"Clear Errors.vi"("error in (no error)"=w74) -> ()  [unwired: 5 in, 2 out]
        }
        frame True {
          # "屏幕可用宽度或高度不满足最小要求，直接最大化即可。"
          n64 = Unbundle By Name(w117) -> ("UserWidth"=w109:i32, "UserHeight"=w110:i32)
          n65 = Divide(x=w115, y=w111) -> (x/y=w108:dbl)
          n66 = Divide(x=w109, y=w110) -> (x/y=w116:dbl)
          n67 = Greater Or Equal?(x=w116, y=w108) -> (x >= y?=w112:bool)
          n68 = case shown="假" w112 {
            tunnel: w118 -> [w126 w139]
            tunnel: [w125 w129] -> w103
            tunnel: [w121 w138] -> w99
            tunnel: w110 -> [_ w136]
            tunnel: [w119 w137] -> w98
            tunnel: w109 -> [w123 w134]
            tunnel: w108 -> [w122 w135]
            tunnel: [w124 w127] -> w102
            tunnel: w107 -> [_ _]
            frame False {
              # "用满宽度"
              n69 = Unbundle By Name(w126) -> ("left"=w125:i32, "top"=w121:i32)
              n70 = Divide(x=w123, y=w122) -> (x/y=w120:dbl)
              n71 = Add(x=w121, y=w120) -> (x+y=w119:dbl)
              n72 = Add(x=w125, y=w123) -> (x+y=w124:i32)
            }
            frame True {
              # "用满高度"
              n73 = Unbundle By Name(w139) -> ("left"=w131:i32, "top"=w138:i32)
              n74 = Multiply(x=w135, y=w136) -> (x*y=w128:dbl)
              n75 = Subtract(x=w134, y=w128) -> (x-y=w133:dbl)
              n76 = Divide(x=w133, y=2.0) -> (x/y=w130:dbl)
              n77 = Add(x=w131, y=w130) -> (x+y=w129:dbl)
              n78 = Add(x=w129, y=w128) -> (x+y=w127:dbl)
              n79 = Add(x=w138, y=w136) -> (x+y=w137:i32)
            }
          }
          n80 = Subtract(x=w103, y=w102) -> (x-y=w101:dbl)
          n81 = Subtract(x=w99, y=w98) -> (x-y=w100:dbl)
          n82 = Bundle By Name(cluster=T26 {"Left"=0, "Top"=0, "Right"=0, "Bottom"=0} ("前面板窗口:前面板边界"), "Left"=w103, "Top"=w99, "Right"=w102, "Bottom"=w98) -> (w113:T26)
          n83 = Bundle By Name(cluster=T25 {"Horizontal"=0, "Vertical"=0} ("前面板窗口:最小尺寸"), "Horizontal"=w101, "Vertical"=w100) -> (w104:T25)
          n84 = property class="VI"(reference=w107, "Minimum Panel Size"=w104) -> (reference out=w106:refnum<vi>)  [unwired: 1 in, 1 out]
          n85 = property class="VI"(reference=w106, "Front Panel.WinBounds"=w113) -> ()  [unwired: 1 in, 2 out]
        }
      }
      n86 = local write "dbcSigOver1"(FALSE ("dbcSigOver1")) -> ()
    }
    frame #1 {
      w158 = FALSE ("可见")
      # "本帧为控件初始化"
      n87 = invoke class="XYGraph (严格)" method="Reinit To Default"(reference=w180) -> ()  [unwired: 2 in, 3 out]
      n88 = property class="Bool (严格)"(reference=w168, "Value"=FALSE ("值")) -> ()  [unwired: 1 in, 2 out]
      n89 = invoke class="Tree (严格)" method="Edit Tree Items.Delete"(reference=w182) -> ()  [unwired: 4 in, 5 out]
      n90 = call "InitParameters.vi"("appended path"=w161) -> ("Settings"=w166:T6, "LastCANpath"=w152:path, "LastDBCpath"=w144:path)  [unwired: 6 in, 1 out]
      n91 = property class="Clust (严格)"(reference=w165, "Value"=w166) -> (reference out=w160:refnum<vi>)  [unwired: 1 in, 1 out]
      n92 = local write "CANpath"(path "" ("值")) -> ()
      n93 = call <vilib>:"Check if File or Folder Exists.vi"("path"=w144) -> ("file or folder exists?"=w143:bool, "dup path"=w141:path)  [unwired: 8 in, 1 out]
      n94 = Unbundle By Name(w166) -> ("LangSet"=w154:u32, "TimeFormat"=w146:u16, "TimeRerange"=w147:bool, "isAutoCurves"=w148:bool, "isAutoY"=w149:bool, "NeedUpdate"=w170:bool, "ChkUpdatePeriod"=w169:u32, "LastTimChkUpdate"=w172:dbl, "NewVersionOnWeb"=w157:string, "LineWidth"=w145:u8, "isShowYValue"=w156:bool, "isShowXY"=w155:bool)
      n95 = control-ref of="txtDrawingPrompt"() -> (w181:refnum<vi>)
      n96 = control-ref of="ProgressNumerical"() -> (w175:refnum<vi>)
      n97 = case shown="真" w143 {
        tunnel: [path "" ("dup path") w188] -> w142
        tunnel: w141 -> [_ w188]
        tunnel: [T27."Disabled and Grayed Out" ("禁用") T27."Enabled" ("禁用")] -> w140
        frame False {
        }
        frame True {
        }
      }
      n98 = local write "LastCANPath"(w152) -> ()
      n99 = control-ref of="SelectedSigList"() -> (w173:refnum<vi>)
      n100 = property class="Str"(reference=w181, "Visible"=w158) -> ()  [unwired: 1 in, 2 out]
      n101 = property on="属性节点" class="MCListbox (严格)"(reference=w173, "ItemNames"=string[][] [] ("项名")) -> ()  [unwired: 1 in, 2 out]
      n102 = property class="Str"(reference=w175, "Visible"=w158) -> ()  [unwired: 1 in, 2 out]
      n103 = control-ref of="XYTips"() -> (w159:refnum<vi>)
      n104 = local write "LineWidth"(w145) -> ()
      n105 = property on="isShowYValue" class="Bool (严格)"("Value"=w156) -> ()  [unwired: 2 in, 2 out]
      n106 = property on="isShowXY" class="Bool (严格)"("Value"=w155) -> ()  [unwired: 2 in, 2 out]
      n107 = property class="Str"(reference=w159, "Visible"=w158) -> ()  [unwired: 1 in, 2 out]
      n108 = control-ref of="HorizontalProgressBar"() -> (w178:refnum<vi>)
      n109 = local write "LastDBCPath"(w142) -> ()
      n110 = property on="boolLoadLastDBC" class="Bool"("DisabledEnum"=w140) -> ()  [unwired: 2 in, 2 out]
      n111 = property class="Slide (严格)"(reference=w178, "Value"=u8 0 ("值")) -> (reference out=w177:refnum<vi>)  [unwired: 1 in, 1 out]
      n112 = local write "TimeFormat"(w146) -> ()
      n113 = local write "isAutoY"(w149) -> ()
      n114 = local write "isTimeRerange"(w147) -> ()
      n115 = local write "isAutoCurves"(w148) -> ()
      n116 = control-ref of="ChkUpdateCnt"() -> (w162:refnum<vi>)
      n117 = call "CompareChkTime.vi"("ChkUpdateCnt"=w162, "LastTimChkUpdate"=w172, "ChkUpdatePeriod"=w169) -> ("OK2Chk"=w171:bool)  [unwired: 8 in]
      n118 = property class="Slide (严格)"(reference=w177, "Visible"=FALSE ("可见")) -> ()  [unwired: 1 in, 2 out]
      n119 = And(x=w171, y=w170) -> (x .and. y?=w164:bool)
      n120 = local write "isDataLoaded"(FALSE ("值")) -> ()
      n121 = case shown="真" w164 {
        tunnel: w154 -> [_ w196]
        tunnel: w157 -> [_ w195]
        tunnel: [0 ("值") w194] -> w163
        tunnel: w161 -> [_ w192]
        tunnel: w160 -> [_ w191]
        tunnel: w157 -> [_ w190]
        frame False {
        }
        frame True {
          n122 = call "VersionCompareIn4Num.vi"("VersionOnWeb"=w195) -> ("realFoundNew"=w193:bool)  [unwired: 10 in]
          n123 = case shown="真" w193 {
            selector: w193 -> [w198 _]
            tunnel: w196 -> [_ w217]
            tunnel: [w200 1 ("值")] -> w194
            tunnel: w192 -> [w199 _]
            tunnel: w191 -> [w197 _]
            tunnel: w190 -> [_ w215]
            frame False {
              n124 = stacked-sequence {
                tunnel: [0 ("值") _] -> w200
                tunnel: w199 -> [w208 _]
                tunnel: w198 -> [w203 w212]
                tunnel: w197 -> [_ w214]
                frame #0 {
                  n125 = call <vilib>:"Open Config Data.vi"("configuration file path"=w208) -> ("error out"=w204:errorcluster, "refnum"=w205:T30)  [unwired: 8 in, 1 out]
                  n126 = call-poly <vilib>:"Read Key.vi"("section"="UpdateSettings", "error in (no error)"=w204, "default value"=w203, "key"="NeedUpdate", "refnum"=w205) -> ("error out"=w201:errorcluster, "refnum out"=w202:T30)  [unwired: 3 in, 2 out]
                  n127 = call <vilib>:"Close Config Data.vi"("error in (no error)"=w201, "refnum"=w202) -> ()  [unwired: 8 in, 2 out]
                }
                frame #1 {
                  n128 = property class="Clust (严格)"(reference=w214) -> (reference out=w210:refnum<vi>, "Value"=w213:T6)  [unwired: 1 in, 1 out]
                  n129 = Bundle By Name(cluster=w213, "NeedUpdate"=w212) -> (w211:T6)
                  n130 = property class="Clust (严格)"(reference=w210, "Value"=w211) -> ()  [unwired: 1 in, 2 out]
                }
              }
            }
            frame True {
              n131 = call "UpdateNowTips.vi"("NewVersionOnWeb"=w215, "LangSet"=w217) -> ("UpdateNow"=w218:bool)  [unwired: 9 in]
              n132 = case shown="真" w218 {
                frame False {
                }
                frame True {
                  n133 = call "RunUpdater.vi"() -> ()  [unwired: 12 in]
                }
              }
            }
          }
        }
      }
      n134 = global write "GlobalVar.vi" "Language"(w154) -> ()
      n135 = control-ref of="GraphLegendWidth"() -> (w184:refnum<vi>)
      n136 = property class="DigNum (严格)"(reference=w184, "Value"=u32 170 ("图例:大小:宽度")) -> ()  [unwired: 1 in, 2 out]
      n137 = property on="Language" class="DigNum (严格)"("Value"=w154) -> ()  [unwired: 2 in, 2 out]
      n138 = local write "NumSelected"(0 ("已选数量")) -> ()
      n139 = property class="DigNum (严格)"(reference=w162, "Value"=w163) -> ()  [unwired: 1 in, 2 out]
    }
    frame #2 {
      w232 = T31 {"Visible"=FALSE, "Color"=12357519, "LineWidth"=2} ("Cursor1")
      w228 = T31 {"Visible"=FALSE, "Color"=1644912, "LineWidth"=2} ("Cursor0")
      w233 = FALSE ("DBC_loaded")
      w251 = 0 ("报文行数")
      # "本帧为变量初始化"
      n140 = control-ref of="ManuCofigofYaxle"() -> (w249:refnum<vi>)
      n141 = property class="Arr (严格)"(reference=w249) -> (reference out=w248:refnum<vi>, "Value"=w247:cluster{"Y轴序号":u8, "Y轴名称":string, "可见性":bool}[])  [unwired: 1 in, 1 out]
      n142 = property class="XYGraph (严格)"(reference=w231, "Active Cursor"=u32 0 ("活动游标")) -> (reference out=w229:refnum<vi>)  [unwired: 1 in, 1 out]
      n143 = property class="Bool (严格)"(reference=w238, "Value"=TRUE ("值")) -> ()  [unwired: 1 in, 2 out]
      n144 = property on="CanMessageRowsNum" class="DigNum (严格)"("Value"=w251) -> ()  [unwired: 2 in, 2 out]
      n145 = Index Array(array=w247, index=0 ("索引")) -> (element=w245:cluster{"Y轴序号":u8, "Y轴名称":string, "可见性":bool})
      n146 = for {
        N: w250 -> [_]
        tunnel: w245 -> [w258]
        tunnel: [w254] -> w244 mode=indexing
        i -> [w257]
        n147 = Increment(x=w257) -> (x+1=w260:i32)
        n148 = Number To Decimal String(number=w260) -> (decimal integer string=w259:string)  [unwired: 1 in]
        n149 = Concatenate Strings("Y", w259) -> (w256:string)
        n150 = Bundle By Name(cluster=w258, "Y轴序号"=w257, "Y轴名称"=w256, "可见性"=TRUE) -> (w254:cluster{"Y轴序号":u8, "Y轴名称":string, "可见性":bool})
      }
      n151 = property on="FileSize" class="DigNum (严格)"("Value"=w251) -> ()  [unwired: 2 in, 2 out]
      n152 = property class="Arr (严格)"(reference=w248, "Value"=w244) -> ()  [unwired: 1 in, 2 out]
      n153 = Unbundle By Name(w228) -> ("Visible"=w220:bool, "Color"=w227:u32, "LineWidth"=w226:u8)
      n154 = global write "GlobalVariables.vi" "Cursor0"(w228) -> ()
      n155 = property on="isAutoCurves" class="Bool (严格)"() -> ("Value"=w236:T5)  [unwired: 2 in, 2 out]
      n156 = property on="isAutoY" class="Bool (严格)"() -> ("Value"=w237:T5)  [unwired: 2 in, 2 out]
      n157 = control-ref of="CurveCustomSealedArray"() -> (w243:refnum<vi>)
      n158 = control-ref of="Language"() -> (w241:refnum<vi>)
      n159 = control-ref of="本VI"() -> (w240:refnum<vi>)
      n160 = property on="CursorTXT1" class="Str"("Visible"=w220) -> ()  [unwired: 2 in, 2 out]
      n161 = property on="CursorNum1" class="DigNum (严格)"("Visible"=w220) -> ()  [unwired: 2 in, 2 out]
      n162 = property class="Arr (严格)"(reference=w243, "Value"=string[][] [] ("值")) -> ()  [unwired: 1 in, 2 out]
      n163 = property class="XYGraph (严格)"(reference=w229, "Cursor.Visible"=w220, "Cursor.Cursor Color"=w227, "Cursor.LineWidth"=w226) -> (reference out=w225:refnum<vi>)  [unwired: 1 in, 1 out]
      n164 = And(x=w237, y=w236) -> (x .and. y?=w234:T5)
      n165 = case shown="假" w234 {
        tunnel: [T27."Enabled" ("禁用") T27."Disabled and Grayed Out" ("禁用")] -> w235
        frame False {
        }
        frame True {
        }
      }
      n166 = property class="XYGraph (严格)"(reference=w225, "Active Cursor"=u32 1 ("活动游标")) -> (reference out=w223:refnum<vi>)  [unwired: 1 in, 1 out]
      n167 = call "UIinit_Main.vi"("VIref"=w240, "Language"=w241) -> ()  [unwired: 10 in]
      n168 = Unbundle By Name(w232) -> ("Visible"=w219:bool, "Color"=w222:u32, "LineWidth"=w221:u8)
      n169 = global write "GlobalVariables.vi" "Cursor1"(w232) -> ()
      n170 = property on="btnConfigYandCurves" class="Bool"("DisabledEnum"=w235) -> ()  [unwired: 2 in, 2 out]
      n171 = property on="CursorTXT2" class="Str"("Visible"=w219) -> ()  [unwired: 2 in, 2 out]
      n172 = property on="CursorNum2" class="DigNum (严格)"("Visible"=w219) -> ()  [unwired: 2 in, 2 out]
      n173 = property class="XYGraph (严格)"(reference=w223, "Cursor.Visible"=w219, "Cursor.Cursor Color"=w222, "Cursor.LineWidth"=w221) -> ()  [unwired: 1 in, 2 out]
      "DBC_loaded" <- w233
      "Data_loaded" <- w233
      "MainGrapgDraw_finished" <- w233
    }
    frame #3 {
      n174 = property class="XYGraph (严格)"(reference=w267, "Active Cursor"=u32 0 ("活动游标"), "Cursor.Visible"=FALSE ("游标.可见")) -> (reference out=w262:refnum<vi>)  [unwired: 1 in, 1 out]
      n175 = property class="XYGraph (严格)"(reference=w262, "Active Cursor"=u32 1 ("活动游标"), "Cursor.Visible"=FALSE ("游标.可见")) -> ()  [unwired: 1 in, 2 out]
      n176 = case shown="真" FALSE {
        tunnel: w267 -> [_ w271]
        tunnel: w269 -> [_ w270]
        frame False {
        }
        frame True {
          n177 = call "AdjustXYLegend.vi"("SelectedSigList"=w270, "XYGraph输入"=w271) -> ()  [unwired: 10 in]
        }
      }
    }
    frame #4 {
      n178 = while {
        tunnel: w278 -> [w290]
        tunnel: w276 -> [w289]
        tunnel: w277 -> [w288]
        tunnel: w280 -> [w287]
        tunnel: w279 -> [w286]
        tunnel: w275 -> [w284]
        tunnel: w274 -> [w283]
        tunnel: w273 -> [w282]
        tunnel: w272 -> [w281]
        stop <- w285 stop-if-true
        n179 = event shown="[7] \"CANpath\": 值改变" {
          selector: _ -> [_ _ _ _ _ _ _ _ _ _ _ _ _ _ _ _ _ _ _ _ _ _ _ _ _ _ _ _ _ _ _ _ _ _ _ _ _ _ _ _ _ _ _ _]
          dyn-events: _ -> [_ _ _ _ _ _ _ _ _ _ _ _ _ _ _ _ _ _ _ _ _ _ _ _ _ _ _ _ _ _ _ _ _ _ _ _ _ _ _ _ _ _ _ _]
          timeout: _ -> [_ _ _ _ _ _ _ _ _ _ _ _ _ _ _ _ _ _ _ _ _ _ _ _ _ _ _ _ _ _ _ _ _ _ _ _ _ _ _ _ _ _ _ _]
          tunnel: ["btnExit" _ _ _ TRUE _ _ _ _ _ _ _ _ _ _ _ _ _ _ _ _ _ _ _ _ _ _ _ _ _ _ _ _ _ _ _ _ _ _ _ _ _ _ _] -> w285
          tunnel: w290 -> [_ _ _ _ _ _ w322 _ _ _ _ _ _ _ _ _ _ _ _ _ w532 _ _ _ _ _ _ _ _ _ _ _ _ _ _ _ _ _ _ _ _ _ _ _]
          tunnel: w289 -> [_ _ _ _ _ _ _ _ _ _ _ _ _ _ _ _ _ _ _ _ w534 _ _ _ _ w655 w723 w726 w745 _ _ _ _ _ _ _ w1120 _ _ w1153 _ _ _ _]
          tunnel: w288 -> [_ _ _ _ _ _ _ _ _ _ _ _ _ _ _ _ _ _ _ w516 _ _ _ _ _ _ _ _ w744 _ _ _ _ _ w1088 _ _ w1122 _ w1155 _ _ _ _]
          tunnel: w287 -> [_ _ _ _ _ _ _ _ _ _ _ _ _ _ _ _ _ _ _ _ w531 _ _ _ _ w656 _ w725 w743 _ _ _ w905 _ _ _ _ _ _ _ _ _ _ _]
          tunnel: w286 -> [_ _ _ _ _ _ _ _ _ _ _ _ _ _ _ _ _ _ _ _ w530 _ _ _ _ w654 _ _ w742 _ _ _ _ _ _ _ _ _ _ _ _ _ _ _]
          tunnel: w284 -> [_ _ _ _ _ _ _ _ _ _ _ _ _ _ _ _ _ _ _ _ _ _ _ _ _ _ _ _ w739 _ _ _ _ _ w1087 _ _ _ _ _ _ _ _ _]
          tunnel: w283 -> [_ _ _ _ _ _ _ _ _ _ _ _ _ _ _ _ _ _ w498 _ _ _ _ _ _ _ _ _ _ _ _ _ _ _ _ _ _ _ _ _ _ _ _ _]
          tunnel: w282 -> [_ _ _ _ _ _ _ _ _ _ _ _ _ _ _ _ _ _ _ _ _ _ _ _ _ _ _ _ _ _ _ _ _ _ _ _ _ _ _ _ _ _ _ _]
          tunnel: w281 -> [_ _ _ _ _ _ _ _ _ _ _ _ _ _ _ _ _ _ _ _ _ _ w551 w598 w638 w659 _ _ _ _ _ w899 _ _ _ _ _ _ _ _ _ _ _ _]
          event Timeout {
            n180 = event-data() -> ()  [unwired: 1 in, 3 out]
          }
          event Value Change {
            n181 = event-data() -> ()  [unwired: 1 in, 6 out]
            n182 = control-ref of="本VI"() -> (w293:refnum<vi>)
            n183 = property class="VI"(reference=w293, "FP.State"=T28."Minimized" ("前面板窗口:状态")) -> ()  [unwired: 1 in, 2 out]
          }
          event Value Change {
            n184 = event-data() -> ("OldVal"=w295:T13)  [unwired: 1 in, 5 out]
            n185 = case shown="假" w295 {
              tunnel: [T28."Standard" ("前面板窗口:状态") T28."Maximized" ("前面板窗口:状态")] -> w294
              frame False {
              }
              frame True {
              }
            }
            n186 = control-ref of="本VI"() -> (w296:refnum<vi>)
            n187 = property class="VI"(reference=w296, "FP.State"=w294) -> ()  [unwired: 1 in, 2 out]
          }
          event Value Change {
            n188 = event-data() -> ()  [unwired: 1 in, 6 out]
            n189 = control-ref of="本VI"() -> (w300:refnum<vi>)
            n190 = call "RunUpdater.vi"("关闭前面板"=FALSE, "VI输入"=w300, "run minimized? (F)"=FALSE) -> ()  [unwired: 9 in]
          }
          event Value Change {
            n191 = event-data() -> ()  [unwired: 1 in, 6 out]
            n192 = control-ref of="本VI"() -> (w304:refnum<vi>)
            n193 = invoke class="VI" method="FP.Close"(reference=w304) -> (reference out=w303:refnum<vi>, error out=w302:errorcluster)  [unwired: 2 in, 1 out]
            n194 = Close Reference(reference=w303, error in (no error)=w302) -> ()  [unwired: 1 out]
          }
          event "boolLoadLastDBC": Mouse Down {
            n195 = event-data() -> ()  [unwired: 1 in, 8 out]
            n196 = global read "GlobalVar.vi" "ConfigIniPath"() -> (w308:path)
            n197 = call <vilib>:"Open Config Data.vi"("configuration file path"=w308) -> ("refnum"=w312:T30)  [unwired: 8 in, 2 out]
            n198 = call-poly <vilib>:"Read Key.vi"("section"="paths", "key"="lastDBCpath", "refnum"=w312) -> ("value"=w307:path, "refnum out"=w309:T30)  [unwired: 5 in, 2 out]
            n199 = call <vilib>:"Close Config Data.vi"("refnum"=w309) -> ()  [unwired: 9 in, 2 out]
            n200 = call <vilib>:"Check if File or Folder Exists.vi"("path"=w307) -> ("file or folder exists?"=w306:bool)  [unwired: 8 in, 2 out]
            n201 = case shown="假" w306 {
              tunnel: w307 -> [_ w313]
              frame False {
                n202 = call "显示对话框信息14"() -> ()  [unwired: 10 in, 2 out]
              }
              frame True {
                n203 = control-ref of="DBCpath"() -> (w314:refnum<vi>)
                n204 = property class="Path"(reference=w314, "Val(Sgnl)"=w313) -> ()  [unwired: 1 in, 2 out]
              }
            }
          }
          event "DBCpath": Value Change {
            n205 = event-data() -> ()  [unwired: 1 in, 6 out]
            n206 = global read "GlobalVar.vi" "ConfigIniPath"() -> (w317:path)
            n207 = local read "DBCpath"() -> (w316:path)
            n208 = Strip Path(path=w316) -> (name=w315:string)  [unwired: 1 out]
            n209 = local write "DBCfileIn"(w315) -> ()
            n210 = call <vilib>:"Open Config Data.vi"("configuration file path"=w317) -> ("refnum"=w319:T30)  [unwired: 8 in, 2 out]
            n211 = call <vilib>:"Get File Extension.vi"("file"=w316) -> ("lowercase file extension"=w320:string, "dup file"=w321:path)  [unwired: 6 in, 3 out]
            n212 = case shown="\"dbc\"" w320 {
              tunnel: w322 -> [_ w327]
              tunnel: w321 -> [_ w325]
              tunnel: w319 -> [w323 w326]
              tunnel: [w323 w324] -> w318
              frame "假", Default {
                n213 = call "显示对话框信息3"() -> ()  [unwired: 10 in, 2 out]
              }
              frame "dbc" {
                n214 = stacked-sequence {
                  tunnel: w327 -> [_ w358 _]
                  tunnel: w326 -> [w341 _ _]
                  tunnel: w325 -> [w338 w354 _]
                  tunnel: [w337 _ _] -> w324
                  frame #0 {
                    w336 = TRUE ("可见")
                    n215 = control-ref of="HorizontalProgressBar"() -> (w335:refnum<vi>)
                    n216 = control-ref of="ProgressNumerical"() -> (w333:refnum<vi>)
                    n217 = control-ref of="txtDrawingPrompt"() -> (w334:refnum<vi>)
                    n218 = call-poly <vilib>:"Write Key.vi"("section"="paths", "value"=w338, "key"="lastDBCpath", "refnum"=w341) -> ("refnum out"=w337:T30)  [unwired: 5 in, 2 out]
                    n219 = property class="Slide (严格)"(reference=w335, "Visible"=w336) -> ()  [unwired: 1 in, 2 out]
                    n220 = property class="Str"(reference=w334, "Visible"=w336) -> (reference out=w331:refnum<vi>)  [unwired: 1 in, 1 out]
                    n221 = global read "GlobalVar.vi" "Language"() -> (w330:u32)
                    n222 = property class="Str"(reference=w333, "Visible"=w336) -> ()  [unwired: 1 in, 2 out]
                    n223 = control-ref of="SelectedSigList"() -> (w342:refnum<vi>)
                    n224 = case shown="409, 默认" w330 {
                      tunnel: ["通叔提示您：程序正在玩命解析DBC，请稍后..." ("key") "Jay Sur tip: the program is playing hard to parse DBC, please wait..." ("key")] -> w332
                      frame 804 {
                      }
                      frame 409, Default {
                      }
                    }
                    n225 = local write "NumSelected"(0 ("值")) -> ()
                    n226 = property on="属性节点" class="MCListbox (严格)"(reference=w342, "ItemNames"=string[][] [] ("项名")) -> ()  [unwired: 1 in, 2 out]
                    n227 = local write "DBC_loaded"(FALSE ("DBC_loaded")) -> ()
                    n228 = property class="Str"(reference=w331, "Value"=w332) -> ()  [unwired: 1 in, 2 out]
                  }
                  frame #1 {
                    # "0-SignalTag\n1-Signal\n2-报文+ID\n3-ID（不带0x的16进制）\n4-起始位\n5-长度\n6-格式\n7-缩放系数\n8-偏移量\n9-最小值\n10-最大值\n11-单位\n12-节点\n13-符号"
                    n229 = control-ref of="AllValueTable"() -> (w357:refnum<vi>)
                    n230 = control-ref of="ProgressNumerical"() -> (w356:refnum<vi>)
                    n231 = control-ref of="HorizontalProgressBar"() -> (w355:refnum<vi>)
                    n232 = call "DBC2Sheet.vi"("进度数值"=w356, "Slide输入"=w355, "DBC树"=w358, "ValueTable"=w357, "file path (dialog if empty)"=w354) -> ("值表数组"=w349:string[][], "信号数"=w348:i32, "数组"=w350:string[][], "报文数"=w347:i32)
                    n233 = local write "CANmessageNum"(w347) -> ()
                    n234 = local write "SigNum"(w348) -> ()
                    n235 = local write "DBCAllSigArry"(w350) -> ()
                    n236 = local write "SigValListArry"(w349) -> ()
                    n237 = Index Array(array=w350, index (col)=0 ("禁用的索引 (列)")) -> (element=w353:string[])  [unwired: 1 in]
                    n238 = Array Size(array=w353) -> (size(s)=w351:i32)
                    n239 = Greater Than 0?(x=w351) -> (x > 0?=w346:bool)
                    n240 = local write "dbcSigOver1"(w346) -> ()
                  }
                  frame #2 {
                    w368 = FALSE ("可见")
                    n241 = control-ref of="HorizontalProgressBar"() -> (w367:refnum<vi>)
                    n242 = control-ref of="txtDrawingPrompt"() -> (w366:refnum<vi>)
                    n243 = control-ref of="ProgressNumerical"() -> (w365:refnum<vi>)
                    n244 = property class="Slide (严格)"(reference=w367, "Visible"=w368) -> ()  [unwired: 1 in, 2 out]
                    n245 = property class="Str"(reference=w366, "Visible"=w368) -> (reference out=w363:refnum<vi>)  [unwired: 1 in, 1 out]
                    n246 = property class="Str"(reference=w365, "Visible"=w368) -> (reference out=w361:refnum<vi>)  [unwired: 1 in, 1 out]
                    n247 = property on="boolLoadLastDBC" class="Bool"("DisabledEnum"=T27."Enabled" ("禁用")) -> ()  [unwired: 2 in, 2 out]
                    n248 = property class="Str"(reference=w361, "Value"="0%" ("值")) -> ()  [unwired: 1 in, 2 out]
                    n249 = property class="Str"(reference=w363, "Value"="" ("key")) -> ()  [unwired: 1 in, 2 out]
                    n250 = local write "DBC_loaded"(TRUE ("DBC_loaded")) -> ()
                  }
                }
              }
            }
            n251 = call <vilib>:"Close Config Data.vi"("refnum"=w318) -> ()  [unwired: 9 in, 2 out]
          }
          event "CANpath": Value Change {
            n252 = event-data() -> ()  [unwired: 1 in, 6 out]
            n253 = stacked-sequence {
              frame #0 {
                w384 = i64 1024 ("y")
                w388 = TRUE ("可见")
                n254 = control-ref of="HorizontalProgressBar"() -> (w379:refnum<vi>)
                n255 = control-ref of="CANpath"() -> (w393:refnum<vi>)
                n256 = local write "Data_loaded"(FALSE ("Data_loaded")) -> ()
                n257 = control-ref of="ProgressNumerical"() -> (w376:refnum<vi>)
                n258 = control-ref of="txtDrawingPrompt"() -> (w392:refnum<vi>)
                n259 = property class="Path"(reference=w393) -> ("Value"=w381:path)  [unwired: 1 in, 2 out]
                n260 = property class="Slide (严格)"(reference=w379, "Value"=u8 0 ("值")) -> (reference out=w378:refnum<vi>)  [unwired: 1 in, 1 out]
                n261 = property class="Str"(reference=w376, "Value"="" ("值")) -> (reference out=w375:refnum<vi>)  [unwired: 1 in, 1 out]
                n262 = Strip Path(path=w381) -> (name=w380:string)  [unwired: 1 out]
                n263 = property on="CANDatafileIn" class="Str"("Value"=w380) -> ()  [unwired: 2 in, 2 out]
                n264 = property class="Slide (严格)"(reference=w378, "Visible"=w388) -> (reference out=w391:refnum<vi>)  [unwired: 1 in, 1 out]
                n265 = control-ref of="CanMessageRowsNum"() -> (w382:refnum<vi>)
                n266 = call <vilib>:"Get File Extension.vi"("file"=w381) -> ("lowercase file extension"=w387:string)  [unwired: 6 in, 4 out]
                n267 = property class="Str"(reference=w375, "Visible"=w388) -> (reference out=w390:refnum<vi>)  [unwired: 1 in, 1 out]
                n268 = property class="Str"(reference=w392, "Visible"=w388) -> (reference out=w389:refnum<vi>)  [unwired: 1 in, 1 out]
                n269 = local read "Language"() -> (w370:u32)
                n270 = Get File Size(file=w381) -> (size (in bytes)=w386:i64)  [unwired: 1 in, 2 out]
                n271 = case shown="\"csv\"" w387 {
                  tunnel: w391 -> [w402 w411 w420 w427 w433 w445 w448]
                  tunnel: w390 -> [w401 w410 w419 w426 w434 w444 w449]
                  tunnel: w389 -> [w400 w409 w418 w428 w430 w446 w456]
                  tunnel: [w399 w408 w417 w429 w437 w447 w454] -> w371
                  tunnel: w381 -> [w398 w407 w416 w425 w431 w443 w451]
                  tunnel: w382 -> [w397 w406 w415 w424 w432 w442 w450]
                  tunnel: [w396 w405 w414 w423 w438 w441 w455] -> w372
                  tunnel: [w395 w404 w413 w422 w436 w440 w453] -> w373
                  tunnel: w370 -> [w394 w403 w412 w421 w435 w439 w452]
                  frame "txt", Default {
                    n272 = call "FiletxtOpen.vi"("Tips"=w400, "Language"=w394, "ProgressBar"=w402, "ProgressNum"=w401, "MessageLinCnt"=w397, "file path (dialog if empty)"=w398) -> ("重构的Data数组"=w399:u32[][], "BaseTimeCluster"=w396:T15, "CAN报文统计"=w395:string[][])  [unwired: 3 out]
                  }
                  frame "csv" {
                    n273 = call "FilecsvOpen.vi"("提示语"=w409, "Language"=w403, "进度条"=w411, "进度数值"=w410, "报文行数统计"=w406, "file path (dialog if empty)"=w407) -> ("重构的Data数组"=w408:u32[][], "基时间簇"=w405:T15, "CAN报文统计"=w404:string[][])  [unwired: 3 out]
                  }
                  frame "xls", "xlsx" {
                    n274 = call "FileExcelOpen.vi"("提示语"=w418, "Language"=w412, "进度条"=w420, "进度数值"=w419, "报文行数统计"=w415, "file path (dialog if empty)"=w416) -> ("重构的Data数组"=w417:u32[][], "基时间簇"=w414:T15, "CAN报文统计"=w413:string[][])  [unwired: 3 out]
                  }
                  frame "can" {
                    n275 = call "FileCanOpen.vi"("提示语"=w428, "Language"=w421, "进度条"=w427, "进度数值"=w426, "报文行数统计"=w424, "file path (dialog if empty)"=w425) -> ("重构的Data数组"=w429:u32[][], "基时间簇"=w423:T15, "CAN报文统计"=w422:string[][])  [unwired: 3 out]
                  }
                  frame "trc" {
                    n276 = call "FileTrcOpen.vi"("提示语"=w430, "Language"=w435, "进度条"=w433, "进度数值"=w434, "报文行数统计"=w432, "file path (dialog if empty)"=w431) -> ("重构的Data数组"=w437:u32[][], "基时间簇"=w438:T15, "CAN报文统计"=w436:string[][])  [unwired: 3 out]
                  }
                  frame "asc" {
                    n277 = call "FileAscOpen.vi"("提示语"=w446, "Language"=w439, "进度条"=w445, "进度数值"=w444, "报文行数统计"=w442, "file path (dialog if empty)"=w443) -> ("重构的Data数组"=w447:u32[][], "基时间簇"=w441:T15, "CAN报文统计"=w440:string[][])  [unwired: 3 out]
                  }
                  frame "blf" {
                    n278 = call "FileBLFOpen.vi"("提示语"=w456, "Language"=w452, "进度条"=w448, "进度数值"=w449, "报文行数统计"=w450, "file path (dialog if empty)"=w451) -> ("重构的Data数组"=w454:u32[][], "基时间簇"=w455:T15, "CAN报文统计"=w453:string[][])  [unwired: 3 out]
                  }
                }
                n279 = Divide(x=w386, y=w384) -> (x/y=w385:dbl)
                n280 = Divide(x=w385, y=w384) -> (x/y=→"FileSize":dbl)
                n281 = local write "CANMessagesAllInfo"(w373) -> ()
                n282 = local write "DataArryOfCANLoaded"(w371) -> ()
                n283 = local write "BaseTimeCluster"(w372) -> ()
              }
              frame #1 {
                w461 = FALSE ("可见")
                n284 = control-ref of="txtDrawingPrompt"() -> (w464:refnum<vi>)
                n285 = control-ref of="ProgressNumerical"() -> (w462:refnum<vi>)
                n286 = control-ref of="HorizontalProgressBar"() -> (w463:refnum<vi>)
                n287 = control-ref of="boolDrawGraph"() -> (w459:refnum<vi>)
                n288 = property class="Slide (严格)"(reference=w463, "Visible"=w461) -> ()  [unwired: 1 in, 2 out]
                n289 = property class="Bool (严格)"(reference=w459, "DisabledEnum"=T27."Enabled" ("禁用")) -> ()  [unwired: 1 in, 2 out]
                n290 = property class="Str"(reference=w462, "Visible"=w461) -> ()  [unwired: 1 in, 2 out]
                n291 = property class="Str"(reference=w464, "Visible"=w461) -> ()  [unwired: 1 in, 2 out]
                n292 = local write "isDataLoaded"(TRUE ("值")) -> ()
                n293 = local write "Data_loaded"(TRUE ("Data_loaded")) -> ()
              }
            }
          }
          event Value Change {
            n294 = event-data() -> ()  [unwired: 1 in, 6 out]
            n295 = global read "GlobalVar.vi" "ConfigIniPath"() -> (w465:path)
            n296 = call <vilib>:"Open Config Data.vi"("configuration file path"=w465) -> ("error out"=w472:errorcluster, "refnum"=w477:T30)  [unwired: 8 in, 1 out]
            n297 = call-poly <vilib>:"Read Key.vi"("section"="paths", "error in (no error)"=w472, "key"="lastDBCpath", "refnum"=w477) -> ("error out"=w473:errorcluster, "value"=w471:path, "refnum out"=w474:T30)  [unwired: 4 in, 1 out]
            n298 = call <vilib>:"Close Config Data.vi"("error in (no error)"=w473, "refnum"=w474) -> ()  [unwired: 8 in, 2 out]
            n299 = Strip Path(path=w471) -> (stripped path=w470:path)  [unwired: 1 out]
            n300 = call "文件对话框3"("start path"=w470, "pattern (all files)"="*.dbc", "pattern label"="DBC File") -> ("selected path"=w467:path, "exists"=w466:bool)  [unwired: 9 in, 2 out]
            n301 = case shown="真" w466 {
              tunnel: w467 -> [_ w478]
              frame False {
              }
              frame True {
                n302 = control-ref of="DBCpath"() -> (w479:refnum<vi>)
                n303 = property class="Path"(reference=w479, "Val(Sgnl)"=w478) -> ()  [unwired: 1 in, 2 out]
              }
            }
          }
          event Value Change {
            n304 = event-data() -> ()  [unwired: 1 in, 6 out]
            n305 = call "文件对话框4"("pattern (all files)"="*.can;*.txt;*.asc;*.csv;*.trc;*.blf;*.xls;*.xlsx", "pattern label"="CAN Data File") -> ("selected path"=w480:path, "exists"=w481:bool)  [unwired: 10 in, 2 out]
            n306 = case shown="真" w481 {
              tunnel: w480 -> [_ w484]
              frame False {
              }
              frame True {
                n307 = control-ref of="CANpath"() -> (w485:refnum<vi>)
                n308 = property class="Path"(reference=w485, "Val(Sgnl)"=w484) -> ()  [unwired: 1 in, 2 out]
              }
            }
          }
          event "btnCANFileInfo": Value Change {
            n309 = event-data() -> ()  [unwired: 1 in, 6 out]
            n310 = control-ref of="CanMessageRowsNum"() -> (w489:refnum<vi>)
            n311 = property class="DigNum (严格)"(reference=w489) -> ("Value"=w487:i32)  [unwired: 1 in, 2 out]
            n312 = global read "GlobalVar.vi" "Language"() -> (w486:u32)
            n313 = Greater Than 0?(x=w487) -> (x > 0?=w488:bool)
            n314 = case shown="真" w488 {
              tunnel: w487 -> [_ _]
              tunnel: w486 -> [w490 w491]
              frame False {
                n315 = case shown="0, 默认" w490 {
                  frame 0, Default {
                    n316 = call "显示对话框信息9"() -> ()  [unwired: 10 in, 2 out]
                  }
                  frame 804 {
                    n317 = call "显示对话框信息5"() -> ()  [unwired: 10 in, 2 out]
                  }
                }
              }
              frame True {
                n318 = control-ref of="DBCAllSigArry"() -> (w492:refnum<vi>)
                n319 = control-ref of="CANpath"() -> (w494:refnum<vi>)
                n320 = control-ref of="CANMessagesAllInfo"() -> (w493:refnum<vi>)
                n321 = call "LookCANFileInfo.vi"("Path输入"=w494, "Language"=w491, "CAN报文统计"=w493, "DBC数组"=w492) -> ()  [unwired: 7 in]
              }
            }
          }
          event "boolMergeFiles": Value Change {
            n322 = event-data() -> ()  [unwired: 1 in, 6 out]
            n323 = call "CANjoiner.vi"() -> ()  [unwired: 12 in]
          }
          event Value Change {
            n324 = event-data() -> ()  [unwired: 1 in, 6 out]
            n325 = call "openCANdb++.vi"() -> ()  [unwired: 12 in]
          }
          event Value Change {
            n326 = event-data() -> ()  [unwired: 1 in, 6 out]
            n327 = call "openCANtest.vi"() -> ()  [unwired: 12 in]
          }
          event Value Change {
            n328 = event-data() -> ()  [unwired: 1 in, 6 out]
            n329 = call "openCANpro.vi"() -> ()  [unwired: 12 in]
          }
          event Value Change {
            n330 = event-data() -> ()  [unwired: 1 in, 6 out]
            n331 = call "openZCANPRO.vi"() -> ()  [unwired: 12 in]
          }
          event Value Change {
            n332 = event-data() -> ()  [unwired: 1 in, 6 out]
            n333 = call "openTSmaster.vi"() -> ()  [unwired: 12 in]
          }
          event Value Change {
            n334 = event-data() -> ()  [unwired: 1 in, 6 out]
            n335 = call "openOrigin.vi"() -> ()  [unwired: 12 in]
          }
          event Value Change {
            n336 = event-data() -> ()  [unwired: 1 in, 6 out]
            n337 = flat-sequence {
              tunnel: w498 -> [w499]
              tunnel: [w499] -> w497
              tunnel: w497 -> [w507]
              tunnel: [w505] -> w496
              tunnel: [w504] -> w495
              tunnel: w496 -> [w512]
              tunnel: w495 -> [w511]
              frame #0 {
                n338 = call "SetUpPanel.vi"("Settings"=w499) -> ()  [unwired: 10 in]
              }
              frame #1 {
                n339 = property class="Clust (严格)"(reference=w507) -> ("Value"=w506:T6)  [unwired: 1 in, 2 out]
                n340 = Unbundle By Name(w506) -> ("LangSet"=w500:u32, "TimeFormat"=w508:u16, "TimeRerange"=w509:bool, "isAutoCurves"=w505:bool, "isAutoY"=w504:bool, "LineWidth"=w503:u8, "isShowYValue"=w501:bool, "isShowXY"=w502:bool)
                n341 = global write "GlobalVar.vi" "Language"(w500) -> ()
                n342 = property on="isShowYValue" class="Bool (严格)"("Value"=w501) -> ()  [unwired: 2 in, 2 out]
                n343 = property on="isShowXY" class="Bool (严格)"("Value"=w502) -> ()  [unwired: 2 in, 2 out]
                n344 = property on="Language" class="DigNum (严格)"("Val(Sgnl)"=w500) -> ()  [unwired: 2 in, 2 out]
                n345 = property on="TimeFormat" class="Ring (严格)"("Val(Sgnl)"=w508) -> ()  [unwired: 2 in, 2 out]
                n346 = property on="LineWidth" class="DigNum (严格)"("Val(Sgnl)"=w503) -> ()  [unwired: 2 in, 2 out]
                n347 = property on="isAutoCurves" class="Bool (严格)"("Value"=w505) -> ()  [unwired: 2 in, 2 out]
                n348 = property on="isAutoY" class="Bool (严格)"("Value"=w504) -> ()  [unwired: 2 in, 2 out]
                n349 = property on="isTimeRerange" class="Bool (严格)"("Value"=w509) -> ()  [unwired: 2 in, 2 out]
              }
              frame #2 {
                n350 = And(x=w512, y=w511) -> (x .and. y?=w513:bool)
                n351 = case shown="假" w513 {
                  tunnel: [T27."Enabled" ("禁用") T27."Disabled and Grayed Out" ("禁用")] -> w510
                  frame False {
                  }
                  frame True {
                  }
                }
                n352 = property on="btnConfigYandCurves" class="Bool"("DisabledEnum"=w510) -> ()  [unwired: 2 in, 2 out]
              }
            }
          }
          event "LineWidth": Value Change {
            n353 = event-data() -> ("NewVal"=w517:u8)  [unwired: 1 in, 5 out]
            n354 = stacked-sequence {
              tunnel: w517 -> [w524 _]
              tunnel: w516 -> [w523 w528]
              frame #0 {
                n355 = control-ref of="ArrySelectedSig"() -> (w520:refnum<vi>)
                n356 = property class="Arr (严格)"(reference=w520) -> ("Value"=w521:string[][])  [unwired: 1 in, 2 out]
                n357 = Index Array(array=w521, index (col)=1 ("禁用的索引 (列)")) -> (element=w519:string[])  [unwired: 1 in]
                n358 = Array Size(array=w519) -> (size(s)=w518:i32)
                n359 = for {
                  N: w518 -> [_]
                  tunnel: w523 -> [w526]
                  tunnel: w524 -> [w525]
                  i -> [w527]
                  n360 = property class="XYGraph (严格)"(reference=w526, "Active Plot"=w527, "Plot.Line Width"=w525) -> ()  [unwired: 1 in, 2 out]
                }
              }
              frame #1 {
                n361 = invoke class="XYGraph (严格)" method="ForceRedraw"(reference=w528) -> ()  [unwired: 2 in, 3 out]
              }
            }
          }
          event "ListOfDBC": Double Click {
            n362 = event-data() -> ("Tag"=w533:string)  [unwired: 1 in, 9 out]
            n363 = control-ref of="NumSelected"() -> (w529:refnum<vi>)
            n364 = call "AddSig2SelList.vi"("NumSelected"=w529, "DBCAllSigArry"=w530, "YaxleNum"=w531, "SelectedSigList"=w534, "Tag"=w533, "TreeControl输入"=w532) -> ()  [unwired: 6 in]
          }
          event "SelectedSigList": Double Click {
            n365 = event-data() -> ("Row"=w539:i32)  [unwired: 1 in, 8 out]
            n366 = control-ref of="NumSelected"() -> (w537:refnum<vi>)
            n367 = control-ref of="ArrySelectedSig"() -> (w543:refnum<vi>)
            n368 = control-ref of="SelectedSigList"() -> (w547:refnum<vi>)
            n369 = property on="属性节点" class="MCListbox (严格)"(reference=w547) -> (reference out=w545:refnum<vi>, "ItemNames"=w546:string[][])  [unwired: 1 in, 1 out]
            n370 = property class="DigNum (严格)"(reference=w537) -> (reference out=w538:refnum<vi>, "Value"=w536:i32)  [unwired: 1 in, 1 out]
            n371 = property class="Arr (严格)"(reference=w543) -> (reference out=w541:refnum<vi>, "Value"=w542:string[][])  [unwired: 1 in, 1 out]
            n372 = Delete From Array(array=w542, index (row)=w539) -> (array with subset deleted=w540:string[][])  [unwired: 2 in, 1 out]
            n373 = Greater Than 0?(x=w536) -> (x > 0?=w535:bool)
            n374 = Delete From Array(array=w546, index (row)=w539) -> (array with subset deleted=w544:string[][])  [unwired: 2 in, 1 out]
            n375 = property class="Arr (严格)"(reference=w541, "Value"=w540) -> ()  [unwired: 1 in, 2 out]
            n376 = case shown="真" w535 {
              tunnel: w536 -> [_ w550]
              tunnel: w538 -> [_ w549]
              frame False {
              }
              frame True {
                n377 = Decrement(x=w550) -> (x-1=w548:i32)
                n378 = property class="DigNum (严格)"(reference=w549, "Value"=w548) -> ()  [unwired: 1 in, 2 out]
              }
            }
            n379 = property on="属性节点" class="MCListbox (严格)"(reference=w545, "ItemNames"=w544) -> ()  [unwired: 1 in, 2 out]
          }
          event "SelectedSigList": Shortcut Menu Selection (User) {
            n380 = event-data() -> ("CtlRef"=w552:refnum<vi>, "ItemTag"=w555:string, "Coords"=w556:T32)  [unwired: 1 in, 5 out]
            n381 = control-ref of="NumSelected"() -> (w554:refnum<vi>)
            n382 = control-ref of="ArrySelectedSig"() -> (w553:refnum<vi>)
            n383 = case shown="\"SelectedSig_Tips\"" w555 {
              tunnel: w556 -> [_ w564 w579 _ _]
              tunnel: w554 -> [_ w562 _ w591 _]
              tunnel: w553 -> [_ w561 _ w592 _]
              tunnel: w552 -> [_ w557 w578 w590 _]
              tunnel: w551 -> [_ _ _ _ w597]
              frame "假", Default {
              }
              frame "SelectedSig_delete" {
                n384 = invoke class="MCListbox (严格)" method="Point To Row Column"(reference=w557, "Point"=w564) -> (reference out=w563:refnum<vi>, "InBounds"=w558:bool, "CellPosition"=w560:T33)  [unwired: 5 in, 4 out]
                n385 = Unbundle By Name(w560) -> ("Row"=w559:i32)
                n386 = case shown="真" w558 {
                  tunnel: w563 -> [_ w577]
                  tunnel: w562 -> [_ w576]
                  tunnel: w561 -> [_ w575]
                  tunnel: w559 -> [_ w574]
                  frame False {
                  }
                  frame True {
                    n387 = property class="Arr (严格)"(reference=w575) -> (reference out=w570:refnum<vi>, "Value"=w571:string[][])  [unwired: 1 in, 1 out]
                    n388 = property on="属性节点" class="MCListbox (严格)"(reference=w577) -> (reference out=w572:refnum<vi>, "ItemNames"=w573:string[][])  [unwired: 1 in, 1 out]
                    n389 = Delete From Array(array=w571, index (row)=w574) -> (array with subset deleted=w569:string[][])  [unwired: 2 in, 1 out]
                    n390 = property class="Arr (严格)"(reference=w570, "Value"=w569) -> ()  [unwired: 1 in, 2 out]
                    n391 = Delete From Array(array=w573, index (row)=w574) -> (array with subset deleted=w568:string[][])  [unwired: 2 in, 1 out]
                    n392 = Index Array(array=w568, index (col)=0 ("禁用的索引 (列)")) -> (element=w566:string[])  [unwired: 1 in]
                    n393 = property on="属性节点" class="MCListbox (严格)"(reference=w572, "ItemNames"=w568) -> ()  [unwired: 1 in, 2 out]
                    n394 = Array Size(array=w566) -> (size(s)=w565:i32)
                    n395 = property class="DigNum (严格)"(reference=w576, "Value"=w565) -> ()  [unwired: 1 in, 2 out]
                  }
                }
              }
              frame "SelectedSig_lookValue" {
                n396 = invoke class="MCListbox (严格)" method="Point To Row Column"(reference=w578, "Point"=w579) -> (reference out=w583:refnum<vi>, "InBounds"=w580:bool, "CellPosition"=w582:T33)  [unwired: 5 in, 4 out]
                n397 = Unbundle By Name(w582) -> ("Row"=w581:i32)
                n398 = case shown="真" w580 {
                  tunnel: w583 -> [_ w585]
                  tunnel: w581 -> [_ _]
                  frame False {
                  }
                  frame True {
                    # "0-SignalTag\n1-Signal\n2-数值\n3-含义"
                    n399 = control-ref of="SigValListArry"() -> (w584:refnum<vi>)
                    n400 = property class="Arr (严格)"(reference=w584) -> ("Value"=w589:string[][])  [unwired: 1 in, 2 out]
                    n401 = property class="MCListbox (严格)"(reference=w585) -> ("ItemNames"=w588:string[][])  [unwired: 1 in, 2 out]
                    n402 = control-ref of="Language"() -> (w586:refnum<vi>)
                    n403 = property on="属性节点" class="DigNum (严格)"(reference=w586) -> ("Value"=w587:u32)  [unwired: 1 in, 2 out]
                    n404 = call "ListSelectedValue.vi"("Language"=w587, "值表数组"=w589, "已选信号列表"=w588) -> ()  [unwired: 8 in, 1 out]
                  }
                }
              }
              frame "SelectedSig_ClcAll" {
                n405 = property on="属性节点" class="MCListbox (严格)"(reference=w590, "ItemNames"=string[][] [] ("项名")) -> ()  [unwired: 1 in, 2 out]
                n406 = property class="DigNum (严格)"(reference=w591, "Value"=0 ("值")) -> ()  [unwired: 1 in, 2 out]
                n407 = property class="Arr (严格)"(reference=w592, "Value"=string[][] [] ("值")) -> ()  [unwired: 1 in, 2 out]
              }
              frame "SelectedSig_Tips" {
                n408 = property class="DigNum (严格)"(reference=w597) -> ("Value"=w596:u32)  [unwired: 1 in, 2 out]
                n409 = case shown="409, 默认" w596 {
                  frame 409, Default {
                    n410 = call "显示对话框信息10"() -> ()  [unwired: 10 in, 2 out]
                  }
                  frame 804 {
                    n411 = call "显示对话框信息7"() -> ()  [unwired: 10 in, 2 out]
                  }
                }
              }
            }
          }
          event "SelectedSigList": Shortcut Menu Activation? {
            n412 = event-data() -> ("MenuRef"=w611:refnum<k9>)  [unwired: 1 in, 6 out]
            n413 = property class="DigNum (严格)"(reference=w598) -> ("Value"=w610:u32)  [unwired: 1 in, 2 out]
            n414 = case shown="804" w610 {
              tunnel: ["Delete" "删除"] -> w604
              tunnel: ["Value Table" "查看值定义"] -> w602
              tunnel: ["Clear All" "清空所有"] -> w606
              tunnel: ["Tips" "提示"] -> w599
              frame 409, Default {
              }
              frame 804 {
              }
            }
            n415 = Set Menu Item Info(7:"SelectedSig_delete", 10:w604, 11:w611) -> (3:w609:refnum<k9>)  [unwired: 4 in, 1 out]
            n416 = Set Menu Item Info(7:"SelectedSig_lookValue", 10:w602, 11:w609) -> (3:w608:refnum<k9>)  [unwired: 4 in, 1 out]
            n417 = Set Menu Item Info(7:"SelectedSig_ClcAll", 10:w606, 11:w608) -> (3:w601:refnum<k9>)  [unwired: 4 in, 1 out]
            n418 = Set Menu Item Info(7:"SelectedSig_Tips", 10:w599, 11:w601) -> ()  [unwired: 4 in, 2 out]
            n419 = event-data() -> ()  [unwired: 2 in, 1 out]
          }
          event "ListOfDBC": Shortcut Menu Activation? {
            n420 = event-data() -> ("CtlRef"=w629:refnum<vi>, "MenuRef"=w632:refnum<k9>, "Coords"=w630:T32)  [unwired: 1 in, 4 out]
            n421 = property class="DigNum (严格)"(reference=w638) -> ("Value"=w643:u32)  [unwired: 1 in, 2 out]
            n422 = invoke class="Tree (严格)" method="Point To Row Column"(reference=w629, "Point"=w630) -> ("InBounds"=w628:bool, "Tag"=w625:string)  [unwired: 6 in, 6 out]
            n423 = case shown="409, 默认" w643 {
              tunnel: ["Select this" "选择此项"] -> w641
              tunnel: ["Tips" "提示"] -> w639
              tunnel: ["Fold/Unfold" "折叠/展开"] -> w636
              tunnel: ["Fold All" "全部折叠"] -> w634
              tunnel: ["Unfold All" "全部展开"] -> w631
              frame 409, Default {
              }
              frame 804 {
              }
            }
            n424 = Empty String/Path?(string/path=w625) -> (empty?=w623:bool)
            n425 = Not(x=w628) -> (.not. x?=w624:bool)
            n426 = Equal?(x=w625, y="TREE_COLUMN_HEADERS") -> (x = y?=w622:bool)
            n427 = Compound Arithmetic op=OR ("复合运算")(w624, w623, w622) -> (w621:bool)
            n428 = Not(x=w621) -> (.not. x?=w627:bool)
            n429 = property on="dbcSigOver1" class="Bool (严格)"() -> ("Value"=w620:bool)  [unwired: 2 in, 2 out]
            n430 = Set Menu Item Info(7:"ListofDBC_Select", 9:w627, 10:w641, 11:w632) -> ()  [unwired: 3 in, 2 out]
            n431 = Set Menu Item Info(7:"ListofDBC_Fold", 9:w627, 10:w636, 11:w632) -> ()  [unwired: 3 in, 2 out]
            n432 = Set Menu Item Info(7:"ListofDBC_FoldAll", 9:w620, 10:w634, 11:w632) -> ()  [unwired: 3 in, 2 out]
            n433 = Set Menu Item Info(7:"ListofDBC_Tips", 10:w639, 11:w632) -> ()  [unwired: 4 in, 2 out]
            n434 = Set Menu Item Info(7:"ListofDBC_UnfoldAll", 9:w620, 10:w631, 11:w632) -> ()  [unwired: 3 in, 2 out]
            n435 = event-data() -> ()  [unwired: 2 in, 1 out]
          }
          event "ListOfDBC": Shortcut Menu Selection (User) {
            n436 = event-data() -> ("CtlRef"=w658:refnum<vi>, "ItemTag"=w660:string, "Coords"=w657:T32)  [unwired: 1 in, 5 out]
            n437 = case shown="\"ListofDBC_Tips\"" w660 {
              tunnel: w659 -> [_ _ _ _ _ w717]
              tunnel: w658 -> [_ w668 w679 w702 w713 _]
              tunnel: w657 -> [_ w667 w678 w703 w714 _]
              tunnel: w656 -> [_ w663 _ _ _ _]
              tunnel: w655 -> [_ w662 _ _ _ _]
              tunnel: w654 -> [_ w661 _ _ _ _]
              frame "假", Default {
              }
              frame "ListofDBC_Select" {
                n438 = invoke class="Tree (严格)" method="Point To Row Column"(reference=w668, "Point"=w667) -> (reference out=w664:refnum<vi>, "InBounds"=w666:bool, "Tag"=w665:string)  [unwired: 6 in, 5 out]
                n439 = case shown="真" w666 {
                  tunnel: w665 -> [_ w674]
                  tunnel: w664 -> [_ w673]
                  tunnel: w663 -> [_ w672]
                  tunnel: w662 -> [_ w671]
                  tunnel: w661 -> [_ w670]
                  frame False {
                  }
                  frame True {
                    n440 = control-ref of="NumSelected"() -> (w669:refnum<vi>)
                    n441 = call "AddSig2SelList.vi"("NumSelected"=w669, "DBCAllSigArry"=w670, "YaxleNum"=w672, "SelectedSigList"=w671, "Tag"=w674, "TreeControl输入"=w673) -> ()  [unwired: 6 in]
                  }
                }
              }
              frame "ListofDBC_Fold" {
                n442 = invoke class="Tree (严格)" method="Point To Row Column"(reference=w679, "Point"=w678) -> (reference out=w676:refnum<vi>, "InBounds"=w677:bool, "Tag"=w675:string)  [unwired: 6 in, 5 out]
                n443 = case shown="真" w677 {
                  tunnel: w676 -> [_ w687]
                  tunnel: w675 -> [_ w684]
                  frame False {
                  }
                  frame True {
                    n444 = invoke class="Tree (严格)" method="Navigate Tree.Get Path"(reference=w687, "tag"=w684) -> (reference out=w683:refnum<vi>, "Navigate Tree:Get Path"=w686:string[])  [unwired: 2 in, 2 out]
                    n445 = Array Size(array=w686) -> (size(s)=w685:i32)
                    n446 = case shown="1, 默认" w685 {
                      tunnel: w684 -> [w688 w699]
                      tunnel: w683 -> [w689 w698]
                      tunnel: [w688 w696] -> w682
                      tunnel: [w694 w697] -> w681
                      tunnel: [w693 FALSE] -> w680
                      frame 1, Default {
                        # "父项"
                        n447 = property class="Tree (严格)"(reference=w689, "Active Item Tag"=w688) -> (reference out=w691:refnum<vi>, error out=w690:errorcluster)  [unwired: 1 in]
                        n448 = property class="Tree (严格)"(reference=w691, error in=w690) -> (reference out=w694:refnum<vi>, "Open?"=w692:bool)  [unwired: 1 out]
                        n449 = Not(x=w692) -> (.not. x?=w693:bool)
                      }
                      frame 2 {
                        # "子项"
                        n450 = invoke class="Tree (严格)" method="Navigate Tree.Get Parent"(reference=w698, "tag"=w699) -> (reference out=w697:refnum<vi>, "Navigate Tree:Get Parent"=w696:string)  [unwired: 2 in, 2 out]
                      }
                    }
                    n451 = invoke class="Tree (严格)" method="Open/Close.Item"(reference=w681, "tag"=w682, "Open"=w680) -> ()  [unwired: 2 in, 5 out]
                  }
                }
              }
              frame "ListofDBC_FoldAll" {
                n452 = invoke class="Tree (严格)" method="Point To Row Column"(reference=w702, "Point"=w703) -> (reference out=w700:refnum<vi>, "InBounds"=w701:bool)  [unwired: 6 in, 6 out]
                n453 = case shown="真" w701 {
                  tunnel: w700 -> [_ w710]
                  frame False {
                  }
                  frame True {
                    n454 = invoke class="Tree (严格)" method="Open/Close.Open/Close All"(reference=w710, "Open"=FALSE) -> (reference out=w708:refnum<vi>)  [unwired: 2 in, 3 out]
                    n455 = property class="Tree (严格)"(reference=w708) -> (reference out=w705:refnum<vi>, "DispItems"=w707:string[])  [unwired: 1 in, 1 out]
                    n456 = Index Array(array=w707, index=0 ("索引")) -> (element=w704:string)
                    n457 = invoke class="Tree (严格)" method="Open/Close.Ensure Visible"(reference=w705, "tag"=w704) -> ()  [unwired: 2 in, 4 out]
                  }
                }
              }
              frame "ListofDBC_UnfoldAll" {
                n458 = invoke class="Tree (严格)" method="Point To Row Column"(reference=w713, "Point"=w714) -> (reference out=w711:refnum<vi>, "InBounds"=w712:bool)  [unwired: 6 in, 6 out]
                n459 = case shown="真" w712 {
                  tunnel: w711 -> [_ w716]
                  frame False {
                  }
                  frame True {
                    n460 = invoke class="Tree (严格)" method="Open/Close.Open/Close All"(reference=w716, "Open"=TRUE) -> ()  [unwired: 2 in, 4 out]
                  }
                }
              }
              frame "ListofDBC_Tips" {
                n461 = property class="DigNum (严格)"(reference=w717) -> ("Value"=w718:u32)  [unwired: 1 in, 2 out]
                n462 = case shown="409, 默认" w718 {
                  frame 409, Default {
                    n463 = call "显示对话框信息11"() -> ()  [unwired: 10 in, 2 out]
                  }
                  frame 804 {
                    n464 = call "显示对话框信息12"() -> ()  [unwired: 10 in, 2 out]
                  }
                }
              }
            }
          }
          event "ClearSelectedSig": Value Change {
            n465 = event-data() -> ()  [unwired: 1 in, 6 out]
            n466 = control-ref of="NumSelected"() -> (w720:refnum<vi>)
            n467 = control-ref of="ArrySelectedSig"() -> (w721:refnum<vi>)
            n468 = property on="属性节点" class="MCListbox (严格)"(reference=w723, "ItemNames"=string[][] [] ("项名")) -> ()  [unwired: 1 in, 2 out]
            n469 = property class="DigNum (严格)"(reference=w720, "Value"=0 ("值")) -> ()  [unwired: 1 in, 2 out]
            n470 = property class="Arr (严格)"(reference=w721, "Value"=string[][] [] ("值")) -> ()  [unwired: 1 in, 2 out]
          }
          event "btnConfigYandCurves": Value Change {
            n471 = event-data() -> ()  [unwired: 1 in, 6 out]
            n472 = property on="属性节点" class="MCListbox (严格)"(reference=w726) -> ("ItemNames"=w731:string[][])  [unwired: 1 in, 2 out]
            n473 = Index Array(array=w731, index (col)=0 ("禁用的索引 (列)")) -> (element=w729:string[])  [unwired: 1 in]
            n474 = Array Size(array=w729) -> (size(s)=w728:i32)
            n475 = Greater Than 0?(x=w728) -> (x > 0?=w727:bool)
            n476 = case shown="真" w727 {
              tunnel: w726 -> [_ w738]
              tunnel: w725 -> [_ w737]
              frame False {
                n477 = call "显示对话框信息"() -> ()  [unwired: 10 in, 2 out]
              }
              frame True {
                n478 = control-ref of="ManuCofigofYaxle"() -> (w736:refnum<vi>)
                n479 = control-ref of="ManuCofigofCurves"() -> (w732:refnum<vi>)
                n480 = control-ref of="CurveCustomSealedArray"() -> (w734:refnum<vi>)
                n481 = control-ref of="Language"() -> (w733:refnum<vi>)
                n482 = control-ref of="NumSelected"() -> (w735:refnum<vi>)
                n483 = call "ConfigYscales.vi"("Language"=w733, "曲线自定义封存数组"=w734, "已选数量"=w735, "Y轴手配"=w736, "Y标尺总数"=w737, "曲线手配"=w732, "已选信号列表"=w738) -> ()  [unwired: 4 in]
              }
            }
          }
          event "boolDrawGraph": Value Change {
            n484 = event-data() -> ()  [unwired: 1 in, 6 out]
            n485 = control-ref of="isDataLoaded"() -> (w741:refnum<vi>)
            n486 = property class="Bool (严格)"(reference=w741) -> ("Value"=w740:bool)  [unwired: 1 in, 2 out]
            n487 = case shown="真" w740 {
              tunnel: w745 -> [_ w752]
              tunnel: w744 -> [_ w756]
              tunnel: w743 -> [_ w755]
              tunnel: w742 -> [_ w749]
              tunnel: w739 -> [_ w754]
              frame False {
                n488 = property on="Language" class="DigNum (严格)"() -> ("Value"=w746:u32)  [unwired: 2 in, 2 out]
                n489 = case shown="409, 默认" w746 {
                  frame 409, Default {
                    n490 = call "显示对话框信息8"() -> ()  [unwired: 10 in, 2 out]
                  }
                  frame 804 {
                    n491 = call "显示对话框信息4"() -> ()  [unwired: 10 in, 2 out]
                  }
                }
              }
              frame True {
                n492 = control-ref of="MporofSelSgs"() -> (w751:refnum<vi>)
                n493 = control-ref of="ArrySelectedSig"() -> (w750:refnum<vi>)
                n494 = property on="Language" class="DigNum (严格)"() -> ("Value"=w753:u32)  [unwired: 2 in, 2 out]
                n495 = control-ref of="SelectedSigValListArry"() -> (w747:refnum<vi>)
                n496 = control-ref of="SigValListArry"() -> (w748:refnum<vi>)
                n497 = call "ListSelectedSigArry.vi"("SelectedSigValListArry"=w747, "已选信号选择器"=w751, "SigValListArry"=w748, "全部信号数组"=w749, "已选信号数组"=w750, "已选列表"=w752) -> ()  [unwired: 5 in, 1 out]
                n498 = stacked-sequence {
                  seq-local: [_ _ _ w852 _ _ _ _] -> [_ _ _ _ w855 _ _ _]
                  tunnel: w756 -> [w767 w775 w812 _ _ w860 w864 w879]
                  tunnel: w750 -> [_ w777 w811 w851 _ _ w862 _]
                  tunnel: w755 -> [_ w776 w810 _ _ _ w863 _]
                  tunnel: w754 -> [_ _ _ _ _ w857 _ _]
                  tunnel: w753 -> [_ w770 w803 w847 _ _ w865 _]
                  tunnel: w751 -> [_ _ _ w844 _ _ _ _]
                  frame #0 {
                    n499 = invoke class="XYGraph (严格)" method="Reinit To Default"(reference=w767) -> (reference out=w766:refnum<vi>)  [unwired: 2 in, 2 out]
                    n500 = property on="Language" class="DigNum (严格)"() -> ("Value"=w758:u32)  [unwired: 2 in, 2 out]
                    n501 = control-ref of="GraphLegendWidth"() -> (w763:refnum<vi>)
                    n502 = case shown="409, 默认" w758 {
                      tunnel: ["Start drawing..." ("值") "开始绘图..." ("值")] -> w759
                      frame 409, Default {
                      }
                      frame 804 {
                      }
                    }
                    n503 = local write "MainGrapgDraw_finished"(FALSE ("MainGrapgDraw_finished")) -> ()
                    n504 = property class="DigNum (严格)"(reference=w763) -> ("Value"=w764:u32)  [unwired: 1 in, 2 out]
                    n505 = control-ref of="txtDrawingPrompt"() -> (w761:refnum<vi>)
                    n506 = property class="Str"(reference=w761, "Value"=w759) -> (reference out=w760:refnum<vi>)  [unwired: 1 in, 1 out]
                    n507 = property class="XYGraph (严格)"(reference=w766, "LegAutosize"=FALSE ("图例:自动调整大小"), "LegWidth"=w764) -> ()  [unwired: 1 in, 2 out]
                    n508 = property class="Str"(reference=w760, "Visible"=TRUE ("可见")) -> ()  [unwired: 1 in, 2 out]
                  }
                  frame #1 {
                    # "所有纵坐标配置"
                    n509 = control-ref of="isAutoY"() -> (w771:refnum<vi>)
                    n510 = property class="Bool (严格)"(reference=w771) -> ("Value"=w772:T34)  [unwired: 1 in, 2 out]
                    n511 = case shown="409, 默认" w770 {
                      tunnel: ["Configurating axis" ("值") "配置坐标轴" ("值")] -> w774
                      frame 409, Default {
                      }
                      frame 804 {
                      }
                    }
                    n512 = case shown="真" w772 {
                      tunnel: w777 -> [_ w801]
                      tunnel: w776 -> [w787 w800]
                      tunnel: w775 -> [w789 w799]
                      frame False {
                        w781 = u8 1
                        n513 = control-ref of="ManuCofigofYaxle"() -> (w790:refnum<vi>)
                        n514 = property class="Arr (严格)"(reference=w790) -> ("Value"=w788:cluster{"Y轴序号":u8, "Y轴名称":string, "可见性":bool}[])  [unwired: 1 in, 2 out]
                        n515 = call "RGBA2U32.vi"("B(0to255)"=u8 189, "G(0to255)"=u8 219, "R(0to255)"=u8 227, "Transparency (0or1)"=u8 0) -> ("ColorU32"=w782:u32)  [unwired: 6 in]
                        n516 = call "RGBA2U32.vi"("B(0to255)"=w781, "G(0to255)"=w781, "R(0to255)"=w781, "Transparency (0or1)"=w781) -> ("ColorU32"=w780:u32)  [unwired: 6 in]
                        n517 = for {
                          N: w787 -> [_]
                          tunnel: w788 -> [w798] mode=indexing
                          tunnel: w789 -> [w797]
                          tunnel: w782 -> [w792]
                          tunnel: w780 -> [w791]
                          n518 = Unbundle By Name(w798) -> ("Y轴序号"=w795:u8, "可见性"=w794:bool, "Y轴名称"=w796:string)
                          n519 = Select(t=w792, s=w794, f=w791) -> (s? t:f=w793:u32)
                          n520 = property class="XYGraph (严格)"(reference=w797, "ActYScl"=w795, "YScale.Visible"=w794, "YScale.MajGrdColor"=w793, "YScale.NameLbl.Text"=w796) -> ()  [unwired: 1 in, 2 out]
                        }
                      }
                      frame True {
                        n521 = call "AutoConfigYScales.vi"("Y标尺总数"=w800, "已选信号数组"=w801, "XYGraph输入"=w799) -> ()  [unwired: 9 in]
                      }
                    }
                    n522 = control-ref of="txtDrawingPrompt"() -> (w773:refnum<vi>)
                    n523 = property class="Str"(reference=w773, "Value"=w774) -> ()  [unwired: 1 in, 2 out]
                  }
                  frame #2 {
                    # "所有曲线配置"
                    n524 = control-ref of="ManuCofigofCurves"() -> (w809:refnum<vi>)
                    n525 = control-ref of="isAutoCurves"() -> (w804:refnum<vi>)
                    n526 = property class="Arr (严格)"(reference=w809) -> ("Value"=w805:T19)  [unwired: 1 in, 2 out]
                    n527 = property class="Bool (严格)"(reference=w804) -> ("Value"=w807:T34)  [unwired: 1 in, 2 out]
                    n528 = property on="LineWidth" class="DigNum (严格)"() -> ("Value"=w802:u8)  [unwired: 2 in, 2 out]
                    n529 = Empty Array?(array=w805) -> (empty?=w808:bool)
                    n530 = Or(x=w807, y=w808) -> (x .or. y?=w806:T34)
                    n531 = case shown="409, 默认" w803 {
                      tunnel: ["Configurating curves' name" ("值") "配置曲线名称" ("值")] -> w814
                      frame 409, Default {
                      }
                      frame 804 {
                      }
                    }
                    n532 = case shown="真" w806 {
                      tunnel: w812 -> [w822 w843]
                      tunnel: w811 -> [w820 w842]
                      tunnel: w810 -> [_ w841]
                      tunnel: w805 -> [w823 _]
                      tunnel: w802 -> [w821 w840]
                      frame False {
                        n533 = property class="Arr (严格)"(reference=w820) -> ("Value"=w819:string[][])  [unwired: 1 in, 2 out]
                        n534 = Index Array(array=w819, index (col)=14 ("禁用的索引 (列)")) -> (element=w817:string[])  [unwired: 1 in]
                        n535 = for {
                          tunnel: w823 -> [w835] mode=indexing
                          tunnel: w822 -> [w834]
                          tunnel: w821 -> [w828]
                          tunnel: w817 -> [w827]
                          n536 = Unbundle By Name(w835) -> ("曲线序号"=w826:u8, "自定义名"=w829:string, "SignalName"=w831:string, "关联Y轴"=w833:u8)
                          n537 = Index Array(array=w827, index=w826) -> (element=w825:string)
                          n538 = case shown="\"1\"" w825 {
                            tunnel: [u8 2 ("曲线.曲线插值") u8 3 ("曲线.曲线插值")] -> w824
                            frame "0", Default {
                            }
                            frame "1" {
                            }
                          }
                          n539 = Empty String/Path?(string/path=w829) -> (empty?=w832:bool)
                          n540 = case shown="假" w832 {
                            tunnel: w831 -> [_ w839]
                            tunnel: [w838 w839] -> w830
                            tunnel: w829 -> [w838 _]
                            frame False {
                            }
                            frame True {
                            }
                          }
                          n541 = property class="XYGraph (严格)"(reference=w834, "Active Plot"=w826, "Plot.Plot Name"=w830, "Plot.YScaleIdx"=w833, "Plot.Line Width"=w828, "Plot.Plot Interpolation"=w824) -> ()  [unwired: 1 in, 2 out]
                        }
                      }
                      frame True {
                        n542 = call "AutoConfigPlots.vi"("LineWidth"=w840, "Y标尺总数"=w841, "已选信号数组"=w842, "XYGraph输入"=w843) -> ()  [unwired: 8 in]
                      }
                    }
                    n543 = control-ref of="txtDrawingPrompt"() -> (w813:refnum<vi>)
                    n544 = property class="Str"(reference=w813, "Value"=w814) -> ()  [unwired: 1 in, 2 out]
                  }
                  frame #3 {
                    n545 = control-ref of="txtDrawingPrompt"() -> (w849:refnum<vi>)
                    n546 = property on="isTimeRerange" class="Bool (严格)"() -> ("Value"=w846:T5)  [unwired: 2 in, 2 out]
                    n547 = control-ref of="DataArryOfCANLoaded"() -> (w848:refnum<vi>)
                    n548 = case shown="409, 默认" w847 {
                      tunnel: ["Drawing lines..." ("值") "绘制曲线..." ("值")] -> w850
                      frame 409, Default {
                      }
                      frame 804 {
                      }
                    }
                    n549 = call "Arry2XYdata.vi"("ClusterSigFormat"="ClusterSigFormat", "MporofSelSgs"=w844, "Value"=w846, "ArrySelectedSig"=w851, "Array输入"=w848) -> ("数组"=w852:cluster{"时间(s)":dbl[], "数据":dbl[]}[])  [unwired: 6 in]
                    n550 = property class="Str"(reference=w849, "Value"=w850) -> ()  [unwired: 1 in, 2 out]
                  }
                  frame #4 {
                    n551 = control-ref of="XYGraphData"() -> (w856:refnum<vi>)
                    n552 = property class="Arr (严格)"(reference=w856, "Value"=w855) -> ()  [unwired: 1 in, 2 out]
                  }
                  frame #5 {
                    n553 = control-ref of="TimeFormat"() -> (w858:refnum<vi>)
                    n554 = control-ref of="XYGraphData"() -> (w859:refnum<vi>)
                    n555 = call "DrawToXYgraph.vi"("BaseTimeCluster"=w857, "XYGraphData"=w859, "TimeFormat"=w858, "XYGraph输入"=w860) -> ()  [unwired: 8 in]
                  }
                  frame #6 {
                    # "读取右侧Y轴的位置和宽度"
                    n556 = case shown="409, 默认" w865 {
                      tunnel: ["Finished!" ("值") "大功告成" ("值")] -> w867
                      frame 409, Default {
                      }
                      frame 804 {
                      }
                    }
                    n557 = control-ref of="txtDrawingPrompt"() -> (w866:refnum<vi>)
                    n558 = call "AutoAdjustYAlxes.vi"("已选信号数组"=w862, "YaxleNum"=w863, "XYGraph输入"=w864) -> ("显示的Y轴数"=w861:i32)  [unwired: 8 in]
                    n559 = property class="Str"(reference=w866, "Value"=w867) -> ()  [unwired: 1 in, 2 out]
                    n560 = property on="Y_DisplayNum" class="DigNum (严格)"("Value"=w861) -> ()  [unwired: 2 in, 2 out]
                  }
                  frame #7 {
                    n561 = control-ref of="本VI"() -> (w878:refnum<vi>)
                    n562 = property class="VI"(reference=w878) -> ("Front Panel.PanelBounds"=w877:T26)  [unwired: 1 in, 2 out]
                    n563 = control-ref of="txtDrawingPrompt"() -> (w883:refnum<vi>)
                    n564 = Unbundle By Name(w877) -> ("Right"=w876:i16, "Left"=w875:i16)
                    n565 = local write "MainGrapgDraw_finished"(TRUE ("MainGrapgDraw_finished")) -> ()
                    n566 = Subtract(x=w876, y=w875) -> (x-y=w874:i16)
                    n567 = property class="Str"(reference=w883, "Visible"=FALSE ("可见")) -> (reference out=w880:refnum<vi>)  [unwired: 1 in, 1 out]
                    n568 = Divide(x=w874, y=i16 9) -> (x/y=w872:dbl)
                    n569 = To Unsigned Long Integer(number=w872) -> (unsigned 32bit integer=w871:u32)
                    n570 = property class="Str"(reference=w880, "Value"="" ("值")) -> ()  [unwired: 1 in, 2 out]
                    n571 = property class="XYGraph (严格)"(reference=w879, "LegWidth"=w871) -> ()  [unwired: 1 in, 2 out]
                  }
                }
              }
            }
          }
          event "MainGraph": Mouse Down {
            n572 = event-data() -> ("CtlRef"=w885:refnum<vi>, "Coords"=w886:T32, "Button"=w884:u16)  [unwired: 1 in, 5 out]
            n573 = control-ref of="ZoomMode"() -> (w887:refnum<vi>)
            n574 = case shown="1" w884 {
              tunnel: w885 -> [_ w889 _ _]
              tunnel: w886 -> [_ w890 _ _]
              tunnel: w887 -> [_ w888 _ _]
              frame 0, Default {
              }
              frame 1 {
                # "左键"
                n575 = call "SetZoomMode.vi"("Coords"=w890, "ZoomMode"=w888, "XYGraph输入"=w889) -> ()  [unwired: 9 in]
              }
              frame 2 {
                # "右键"
              }
              frame 3 {
                # "中键"
              }
            }
          }
          event "MainGraph": Mouse Wheel {
            n576 = event-data() -> ("CtlRef"=w896:refnum<vi>, "Coords"=w895:T32, "Delta"=w894:i32, "PlatMods"=w893:T35)  [unwired: 1 in, 6 out]
            n577 = local read "Y_DisplayNum"() -> (w891:i32)
            n578 = local read "ZoomMode"() -> (w892:u16)
            n579 = call "MouseScrollAction.vi"("XYGraph输入"=w896, "Ynum"=w891, "Coords"=w895, "Delta"=w894, "PlatMods"=w893, "ZoomMode"=w892) -> ()  [unwired: 14 in]
          }
          event "MainGraph": Shortcut Menu Activation? {
            n580 = event-data() -> ("CtlRef"=w900:refnum<vi>, "MenuRef"=w901:refnum<k9>, "Coords"=w902:T32)  [unwired: 1 in, 4 out]
            n581 = property on="isShowYValue" class="Bool (严格)"() -> ("Value"=w898:T5)  [unwired: 2 in, 2 out]
            n582 = property on="isShowXY" class="Bool (严格)"() -> ("Value"=w897:T5)  [unwired: 2 in, 2 out]
            n583 = call "CreateGraphRightKeyMenu.vi"("isFloatXY"=w897, "isShowYvalue"=w898, "Language"=w899, "Coords"=w902, "MenuRef"=w901, "XYGraph输入"=w900) -> ()  [unwired: 6 in]
            n584 = event-data() -> ()  [unwired: 2 in, 1 out]
          }
          event "MainGraph": Shortcut Menu Selection (User) {
            n585 = event-data() -> ("CtlRef"=w904:refnum<vi>, "ItemTag"=w906:string)  [unwired: 1 in, 6 out]
            n586 = control-ref of="Y_DisplayNum"() -> (w903:refnum<vi>)
            n587 = case shown="\"MG_Cursor0_LineWidth\"" w906 {
              tunnel: w905 -> [_ _ _ _ _ _ _ _ _ _ _ _ _ _ _ _ _]
              tunnel: w904 -> [_ _ _ w930 w942 w953 w960 w971 w976 w982 _ w1031 w1042 w1044 w1061 w1069 w1073]
              tunnel: w903 -> [_ _ _ w926 w941 w954 _ _ _ _ _ _ _ _ _ _ _]
              frame "假", Default {
              }
              frame "MainGraph_FloatXY" {
                n588 = global read "GlobalVar.vi" "ConfigIniPath"() -> (w907:path)
                n589 = property on="isShowXY" class="Bool (严格)"() -> ("Value"=w915:T5)  [unwired: 2 in, 2 out]
                n590 = Not(x=w915) -> (.not. x?=w910:T5)
                n591 = call <vilib>:"Open Config Data.vi"("configuration file path"=w907) -> ("error out"=w912:errorcluster, "refnum"=w911:T30)  [unwired: 8 in, 1 out]
                n592 = property on="isShowXY" class="Bool (严格)"("Value"=w910) -> ()  [unwired: 2 in, 2 out]
                n593 = call-poly <vilib>:"Write Key.vi"("section"="DrawSettings", "error in (no error)"=w912, "value"=w910, "key"="isShowXY", "refnum"=w911) -> ("error out"=w908:errorcluster, "refnum out"=w909:T30)  [unwired: 4 in, 1 out]
                n594 = call <vilib>:"Close Config Data.vi"("error in (no error)"=w908, "refnum"=w909) -> ()  [unwired: 8 in, 2 out]
              }
              frame "MainGraph_ShowYvalue" {
                n595 = global read "GlobalVar.vi" "ConfigIniPath"() -> (w916:path)
                n596 = property on="isShowYValue" class="Bool (严格)"() -> ("Value"=w924:T5)  [unwired: 2 in, 2 out]
                n597 = Not(x=w924) -> (.not. x?=w919:T5)
                n598 = call <vilib>:"Open Config Data.vi"("configuration file path"=w916) -> ("error out"=w921:errorcluster, "refnum"=w920:T30)  [unwired: 8 in, 1 out]
                n599 = property on="isShowYValue" class="Bool (严格)"("Value"=w919) -> ()  [unwired: 2 in, 2 out]
                n600 = call-poly <vilib>:"Write Key.vi"("section"="DrawSettings", "error in (no error)"=w921, "value"=w919, "key"="isShowYValue", "refnum"=w920) -> ("error out"=w917:errorcluster, "refnum out"=w918:T30)  [unwired: 4 in, 1 out]
                n601 = call <vilib>:"Close Config Data.vi"("error in (no error)"=w917, "refnum"=w918) -> ()  [unwired: 8 in, 2 out]
              }
              frame "MainGraph_GridDefaults" {
                n602 = property class="DigNum (严格)"(reference=w926) -> ("Value"=w925:i32)  [unwired: 1 in, 2 out]
                n603 = property class="XYGraph (严格)"(reference=w930) -> (reference out=w929:refnum<vi>, "ActYScl"=w927:i32)  [unwired: 1 in, 1 out]
                n604 = for {
                  N: w925 -> [_]
                  tunnel: w929 -> [w934]
                  tunnel: [w931] -> w928
                  i -> [w933]
                  n605 = property class="XYGraph (严格)"(reference=w934, "ActYScl"=w933) -> (reference out=w931:refnum<vi>, "YScale.Visible"=w932:bool)  [unwired: 1 in, 1 out]
                  n606 = case shown="真" w932 {
                    tunnel: w931 -> [_ w935]
                    frame False {
                    }
                    frame True {
                      n607 = call "RGBA2U32.vi"("B(0to255)"=u8 189, "G(0to255)"=u8 219, "R(0to255)"=u8 227, "Transparency (0or1)"=u8 0) -> ("ColorU32"=w936:u32)  [unwired: 6 in]
                      n608 = property class="XYGraph (严格)"(reference=w935, "YScale.MajGrdColor"=w936, "XScale.MajGrdColor"=w936) -> ()  [unwired: 1 in, 2 out]
                    }
                  }
                }
                n609 = property class="XYGraph (严格)"(reference=w928, "ActYScl"=w927) -> ()  [unwired: 1 in, 2 out]
              }
              frame "MainGraph_GridDisableAll" {
                n610 = property class="DigNum (严格)"(reference=w941) -> ("Value"=w945:i32)  [unwired: 1 in, 2 out]
                n611 = property class="XYGraph (严格)"(reference=w942) -> (reference out=w944:refnum<vi>, "BG Color"=w943:u32)  [unwired: 1 in, 1 out]
                n612 = for {
                  N: w945 -> [_]
                  tunnel: w944 -> [w950]
                  tunnel: w943 -> [w946]
                  i -> [w948]
                  n613 = property class="XYGraph (严格)"(reference=w950, "ActYScl"=w948) -> (reference out=w947:refnum<vi>, "YScale.Visible"=w949:bool)  [unwired: 1 in, 1 out]
                  n614 = case shown="真" w949 {
                    tunnel: w947 -> [_ w952]
                    tunnel: w946 -> [_ w951]
                    frame False {
                    }
                    frame True {
                      n615 = property class="XYGraph (严格)"(reference=w952, "YScale.MajGrdColor"=w951, "XScale.MajGrdColor"=w951) -> ()  [unwired: 1 in, 2 out]
                    }
                  }
                }
              }
              frame "MainGraph_ColorPad" {
                n616 = call "ColorSelector.vi"() -> ("颜色"=w955:u32)  [unwired: 11 in]
                n617 = property class="DigNum (严格)"(reference=w954) -> ("Value"=w956:i32)  [unwired: 1 in, 2 out]
                n618 = for {
                  N: w956 -> [_]
                  tunnel: w953 -> [w959]
                  tunnel: w955 -> [w957]
                  i -> [w958]
                  n619 = property class="XYGraph (严格)"(reference=w959, "ActYScl"=w958, "YScale.MajGrdColor"=w957, "XScale.MajGrdColor"=w957) -> ()  [unwired: 1 in, 2 out]
                }
              }
              frame "Graph_CopyYFormats" {
                # "复制Y轴上下限"
                n620 = property class="XYGraph (严格)"(reference=w960) -> (reference out=w965:refnum<vi>, error out=w964:errorcluster, "YScale.Maximum"=w967:dbl, "YScale.Minimum"=w968:dbl, "YScale.NameLbl.Text"=w962:string)  [unwired: 1 in]
                n621 = global read "GlobalVariables.vi" "YFormatsCopy"() -> (w970:T36)
                n622 = property class="XYGraph (严格)"(reference=w965, error in=w964) -> ("ActYScl"=w963:i32)  [unwired: 2 out]
                n623 = Unbundle By Name(w970) -> ("Ylimits"=w969:cluster{"Upbound":dbl, "Downbound":dbl})
                n624 = Bundle(cluster=w969, "Upbound"=w967, "Downbound"=w968) -> (w966:cluster{"Upbound":dbl, "Downbound":dbl})
                n625 = Bundle(cluster=w970, "Ylimits"=w966, "ParentScaleID"=w963, "LabelTitle"=w962) -> (w961:T36)
                n626 = global write "GlobalVariables.vi" "YFormatsCopy"(w961) -> ()
              }
              frame "Graph_PasteY_Limits" {
                # "粘贴Y轴上下限"
                n627 = global read "GlobalVariables.vi" "YFormatsCopy"() -> (w975:T36)
                n628 = Unbundle By Name(w975) -> ("Ylimits"=w974:cluster{"Upbound":dbl, "Downbound":dbl})
                n629 = Unbundle By Name(w974) -> ("Upbound"=w973:dbl, "Downbound"=w972:dbl)
                n630 = property class="XYGraph (严格)"(reference=w971, "YScale.Maximum"=w973, "YScale.Minimum"=w972) -> ()  [unwired: 1 in, 2 out]
              }
              frame "Graph_PasteY_All" {
                # "粘贴Y轴上下限"
                n631 = global read "GlobalVariables.vi" "YFormatsCopy"() -> (w981:T36)
                n632 = Unbundle By Name(w981) -> ("Ylimits"=w980:cluster{"Upbound":dbl, "Downbound":dbl}, "LabelTitle"=w977:string)
                n633 = Unbundle By Name(w980) -> ("Upbound"=w979:dbl, "Downbound"=w978:dbl)
                n634 = property class="XYGraph (严格)"(reference=w976, "YScale.Maximum"=w979, "YScale.Minimum"=w978, "YScale.NameLbl.Text"=w977) -> ()  [unwired: 1 in, 2 out]
              }
              frame "Graph_PasteY_Label" {
                # "粘贴Y轴上下限"
                n635 = global read "GlobalVariables.vi" "YFormatsCopy"() -> (w984:T36)
                n636 = Unbundle By Name(w984) -> ("LabelTitle"=w983:string)
                n637 = property class="XYGraph (严格)"(reference=w982, "YScale.NameLbl.Text"=w983) -> ()  [unwired: 1 in, 2 out]
              }
              frame "MainGraph_Export2CSV" {
                n638 = flat-sequence {
                  tunnel: [w993] -> w990
                  tunnel: [w992] -> w989
                  tunnel: [w991] -> w988
                  tunnel: w990 -> [w1003]
                  tunnel: w989 -> [w1000]
                  tunnel: w988 -> [w1001]
                  tunnel: [w1000] -> w987
                  tunnel: [w1001] -> w986
                  tunnel: [w1002] -> w985
                  tunnel: w987 -> [w1013]
                  tunnel: w986 -> [w1012]
                  tunnel: w985 -> [w1010]
                  frame #0 {
                    w997 = TRUE ("可见")
                    n639 = control-ref of="txtDrawingPrompt"() -> (w996:refnum<vi>)
                    n640 = control-ref of="ProgressNumerical"() -> (w994:refnum<vi>)
                    n641 = control-ref of="HorizontalProgressBar"() -> (w995:refnum<vi>)
                    n642 = property class="Slide (严格)"(reference=w995, "Visible"=w997) -> (reference out=w992:refnum<vi>)  [unwired: 1 in, 1 out]
                    n643 = property class="Str"(reference=w994, "Visible"=w997) -> (reference out=w991:refnum<vi>)  [unwired: 1 in, 1 out]
                    n644 = property class="Str"(reference=w996, "Visible"=w997) -> (reference out=w993:refnum<vi>)  [unwired: 1 in, 1 out]
                  }
                  frame #1 {
                    n645 = control-ref of="ArrySelectedSig"() -> (w1007:refnum<vi>)
                    n646 = control-ref of="MainGraph"() -> (w1008:refnum<vi>)
                    n647 = property class="XYGraph (严格)"(reference=w1008) -> ("Value"=w999:cluster{"时间(s)":dbl[], "数据":dbl[]}[])  [unwired: 1 in, 2 out]
                    n648 = property class="Arr (严格)"(reference=w1007) -> ("Value"=w1006:string[][])  [unwired: 1 in, 2 out]
                    n649 = property class="Str"(reference=w1003, "Value"="通叔提示您：正在导出至CSV，请稍后..." ("key")) -> (reference out=w1002:refnum<vi>)  [unwired: 1 in, 1 out]
                    n650 = Index Array(array=w1006, index (col)=1 ("禁用的索引 (列)")) -> (element=w998:string[])  [unwired: 1 in]
                    n651 = call "Export2CSV.vi"("进度数值"=w1001, "Slide输入"=w1000, "波形数组"=w999, "信号名数组"=w998) -> ()  [unwired: 8 in]
                  }
                  frame #2 {
                    w1014 = FALSE ("可见")
                    n652 = property class="Str"(reference=w1010, "Value"="" ("值")) -> (reference out=w1009:refnum<vi>)  [unwired: 1 in, 1 out]
                    n653 = property class="Slide (严格)"(reference=w1013, "Visible"=w1014) -> ()  [unwired: 1 in, 2 out]
                    n654 = property class="Str"(reference=w1012, "Visible"=w1014) -> ()  [unwired: 1 in, 2 out]
                    n655 = property class="Str"(reference=w1009, "Visible"=w1014) -> ()  [unwired: 1 in, 2 out]
                  }
                }
              }
              frame "MG_Cursor0_Visible" {
                w1026 = u32 0 ("活动游标")
                n656 = control-ref of="CursorNum1"() -> (w1029:refnum<vi>)
                n657 = property class="XYGraph (严格)"(reference=w1031, "Active Cursor"=w1026) -> (reference out=w1021:refnum<vi>, "XScale.Maximum"=w1018:dbl, "XScale.Minimum"=w1019:dbl)  [unwired: 1 in, 1 out]
                n658 = global read "GlobalVariables.vi" "Cursor0"() -> (w1035:T31)
                n659 = control-ref of="CursorTXT1"() -> (w1030:refnum<vi>)
                n660 = Unbundle By Name(w1035) -> ("Visible"=w1036:bool, "Color"=w1033:u32, "LineWidth"=w1032:u8)
                n661 = Add(x=w1018, y=w1019) -> (x+y=w1017:dbl)
                n662 = Divide(x=w1017, y=2.0) -> (x/y=w1015:dbl)
                n663 = property class="XYGraph (严格)"(reference=w1021, "Cursor.Cursor X"=w1015) -> (reference out=w1020:refnum<vi>)  [unwired: 1 in, 1 out]
                n664 = Not(x=w1036) -> (.not. x?=w1028:bool)
                n665 = Bundle By Name(cluster=w1035, "Visible"=w1028, "Color"=w1033, "LineWidth"=w1032) -> (w1034:T31)
                n666 = property class="Str"(reference=w1030, "Visible"=w1028) -> (reference out=w1024:refnum<vi>)  [unwired: 1 in, 1 out]
                n667 = property class="DigNum (严格)"(reference=w1029, "Visible"=w1028) -> (reference out=w1027:refnum<vi>)  [unwired: 1 in, 1 out]
                n668 = property class="XYGraph (严格)"(reference=w1020, "Cursor.Visible"=w1028) -> (reference out=w1025:refnum<vi>, "Cursor.Cursor Position"=w1023:T37)  [unwired: 1 in, 1 out]
                n669 = global write "GlobalVariables.vi" "Cursor0"(w1034) -> ()
                n670 = call "游标移动显示.vi"("偏移值"=-1, "游标位置"=w1023, "CursIdx"=w1026, "游标文本"=w1024, "XYGraph"=w1025, "YBNum"=w1027) -> ()  [unwired: 6 in]
                n671 = case shown="真" w1028 {
                  tunnel: w1025 -> [_ w1038]
                  frame False {
                  }
                  frame True {
                    n672 = property class="XYGraph (严格)"(reference=w1038, "ActPaletteTool"=0 ("选板:活动工具")) -> ()  [unwired: 1 in, 2 out]
                  }
                }
              }
              frame "MG_Cursor0_Color" {
                n673 = property class="XYGraph (严格)"(reference=w1042, "Active Cursor"=u32 0 ("活动游标")) -> (reference out=w1040:refnum<vi>)  [unwired: 1 in, 1 out]
                n674 = call "ColorSelector.vi"() -> ("颜色"=w1039:u32)  [unwired: 11 in]
                n675 = property class="XYGraph (严格)"(reference=w1040, "Cursor.Cursor Color"=w1039) -> ()  [unwired: 1 in, 2 out]
              }
              frame "MG_Cursor0_LineWidth" {
                n676 = call "修改游标线宽.vi"("活动游标"=u32 0, "XYGraph输入"=w1044) -> ()  [unwired: 10 in]
              }
              frame "MG_Cursor1_Visible" {
                w1058 = u32 1 ("活动游标")
                n677 = property class="XYGraph (严格)"(reference=w1061, "Active Cursor"=w1058) -> (reference out=w1047:refnum<vi>, "XScale.Maximum"=w1051:dbl, "XScale.Minimum"=w1050:dbl)  [unwired: 1 in, 1 out]
                n678 = control-ref of="CursorTXT2"() -> (w1060:refnum<vi>)
                n679 = global read "GlobalVariables.vi" "Cursor1"() -> (w1065:T31)
                n680 = control-ref of="CursorNum2"() -> (w1057:refnum<vi>)
                n681 = Add(x=w1051, y=w1050) -> (x+y=w1049:dbl)
                n682 = Divide(x=w1049, y=2.0) -> (x/y=w1045:dbl)
                n683 = Unbundle By Name(w1065) -> ("Visible"=w1066:bool, "Color"=w1063:u32, "LineWidth"=w1062:u8)
                n684 = property class="XYGraph (严格)"(reference=w1047, "Cursor.Cursor X"=w1045) -> (reference out=w1046:refnum<vi>)  [unwired: 1 in, 1 out]
                n685 = Not(x=w1066) -> (.not. x?=w1056:bool)
                n686 = property class="Str"(reference=w1060, "Visible"=w1056) -> (reference out=w1059:refnum<vi>)  [unwired: 1 in, 1 out]
                n687 = Bundle By Name(cluster=w1065, "Visible"=w1056, "Color"=w1063, "LineWidth"=w1062) -> (w1064:T31)
                n688 = property class="DigNum (严格)"(reference=w1057, "Visible"=w1056) -> (reference out=w1055:refnum<vi>)  [unwired: 1 in, 1 out]
                n689 = property class="XYGraph (严格)"(reference=w1046, "Cursor.Visible"=w1056) -> (reference out=w1054:refnum<vi>, "Cursor.Cursor Position"=w1053:T37)  [unwired: 1 in, 1 out]
                n690 = global write "GlobalVariables.vi" "Cursor1"(w1064) -> ()
                n691 = case shown="真" w1056 {
                  tunnel: w1054 -> [_ w1068]
                  frame False {
                  }
                  frame True {
                    n692 = property class="XYGraph (严格)"(reference=w1068, "ActPaletteTool"=0 ("选板:活动工具")) -> ()  [unwired: 1 in, 2 out]
                  }
                }
                n693 = call "游标移动显示.vi"("偏移值"=0, "游标位置"=w1053, "CursIdx"=w1058, "游标文本"=w1059, "XYGraph"=w1054, "YBNum"=w1055) -> ()  [unwired: 6 in]
              }
              frame "MG_Cursor1_Color" {
                n694 = property class="XYGraph (严格)"(reference=w1069, "Active Cursor"=u32 1 ("活动游标")) -> (reference out=w1071:refnum<vi>)  [unwired: 1 in, 1 out]
                n695 = call "ColorSelector.vi"() -> ("颜色"=w1070:u32)  [unwired: 11 in]
                n696 = property class="XYGraph (严格)"(reference=w1071, "Cursor.Cursor Color"=w1070) -> ()  [unwired: 1 in, 2 out]
              }
              frame "MG_Cursor1_LineWidth" {
                n697 = call "修改游标线宽.vi"("活动游标"=u32 1, "XYGraph输入"=w1073) -> ()  [unwired: 10 in]
              }
            }
          }
          event "MainGraph": Cursor Move {
            n698 = event-data() -> ("CtlRef"=w1080:refnum<vi>, "CursIdx"=w1079:i32, "CursLoc"=w1077:cluster{"X":dbl, "Y":dbl})  [unwired: 1 in, 6 out]
            n699 = case shown="1" w1079 {
              tunnel: [w1083 w1084] -> w1078
              tunnel: [w1082 w1085] -> w1076
              tunnel: [-1 ("偏移值") 0 ("偏移值")] -> w1075
              frame 0, Default {
                n700 = control-ref of="CursorNum1"() -> (w1082:refnum<vi>)
                n701 = control-ref of="CursorTXT1"() -> (w1083:refnum<vi>)
              }
              frame 1 {
                n702 = control-ref of="CursorNum2"() -> (w1085:refnum<vi>)
                n703 = control-ref of="CursorTXT2"() -> (w1084:refnum<vi>)
              }
            }
            n704 = call "游标移动显示.vi"("偏移值"=w1075, "游标位置"=w1077, "CursIdx"=w1079, "游标文本"=w1078, "XYGraph"=w1080, "YBNum"=w1076) -> ()  [unwired: 6 in]
          }
          event "TimeFormat": Value Change {
            n705 = event-data() -> ("NewVal"=w1089:u16)  [unwired: 1 in, 5 out]
            n706 = stacked-sequence {
              tunnel: w1089 -> [w1093 w1110]
              tunnel: w1088 -> [w1095 w1109]
              tunnel: w1087 -> [w1094 _]
              frame #0 {
                n707 = control-ref of="XYGraphData"() -> (w1096:refnum<vi>)
                n708 = property class="Clust (严格)"(reference=w1094) -> ("Value"=w1097:T15)  [unwired: 1 in, 2 out]
                n709 = property class="Arr (严格)"(reference=w1096) -> ("Value"=w1092:cluster{"时间(s)":dbl[], "数据":dbl[]}[])  [unwired: 1 in, 2 out]
                n710 = Unbundle By Name(w1097) -> ("基时间秒"=w1091:dbl)
                n711 = case shown="0, 默认" w1093 {
                  tunnel: [w1098 w1100] -> w1090
                  tunnel: w1092 -> [w1098 w1101]
                  tunnel: w1091 -> [_ w1099]
                  frame 0, Default {
                  }
                  frame 1, 2 {
                    n712 = for {
                      tunnel: w1101 -> [w1107] mode=indexing
                      tunnel: [w1106] -> w1100 mode=indexing
                      tunnel: w1099 -> [w1104]
                      n713 = Unbundle(w1107) -> ("时间(s)"=w1103:dbl[], "数据"=w1105:dbl[])
                      n714 = Add(x=w1103, y=w1104) -> (x+y=w1102:dbl[])
                      n715 = Bundle(w1102, "数据"=w1105) -> (w1106:cluster{dbl[], "数据":dbl[]})  [unwired: 1 in]
                    }
                  }
                }
                n716 = property class="XYGraph (严格)"(reference=w1095, "Value"=w1090) -> ()  [unwired: 1 in, 2 out]
              }
              frame #1 {
                n717 = case shown="2" w1110 {
                  tunnel: ["%#.4f" ("X标尺.格式字符串") "%<%H:%M:%S%#.3u>T" ("X标尺.格式字符串") "%<%H:%M:%S%#.3u\n%Y-%m-%d>T" ("X标尺.格式字符串")] -> w1108
                  frame 0, Default {
                  }
                  frame 1 {
                  }
                  frame 2 {
                  }
                }
                n718 = property class="XYGraph (严格)"(reference=w1109, "XScale.FormatString"=w1108) -> ()  [unwired: 1 in, 2 out]
              }
            }
          }
          event "LookAllSigDefinition": Value Change {
            n719 = event-data() -> ()  [unwired: 1 in, 6 out]
            n720 = control-ref of="SigValListArry"() -> (w1115:refnum<vi>)
            n721 = property on="Language" class="DigNum (严格)"() -> ("Value"=w1114:u32)  [unwired: 2 in, 2 out]
            n722 = property class="Arr (严格)"(reference=w1115) -> ("Value"=w1116:string[][])  [unwired: 1 in, 2 out]
            n723 = call "ListAllValue.vi"("Language"=w1114, "值表数组"=w1116) -> ()  [unwired: 9 in, 1 out]
          }
          event "LookSelSigDefinition": Value Change {
            # "0-SignalTag\n1-Signal\n2-数值\n3-含义"
            n724 = event-data() -> ()  [unwired: 1 in, 6 out]
            n725 = control-ref of="SigValListArry"() -> (w1117:refnum<vi>)
            n726 = property class="Arr (严格)"(reference=w1117) -> ("Value"=w1121:string[][])  [unwired: 1 in, 2 out]
            n727 = property class="MCListbox (严格)"(reference=w1120) -> ("ItemNames"=w1119:string[][])  [unwired: 1 in, 2 out]
            n728 = property on="Language" class="DigNum (严格)"() -> ("Value"=w1118:u32)  [unwired: 2 in, 2 out]
            n729 = call "ListSelectedValue.vi"("Language"=w1118, "值表数组"=w1121, "已选信号列表"=w1119) -> ()  [unwired: 8 in, 1 out]
          }
          event "ClearMainGraph": Value Change {
            n730 = event-data() -> ()  [unwired: 1 in, 6 out]
            n731 = invoke class="XYGraph (严格)" method="Reinit To Default"(reference=w1122) -> ()  [unwired: 2 in, 3 out]
          }
          event "boolExport2Excel": Value Change {
            n732 = event-data() -> ()  [unwired: 1 in, 6 out]
            n733 = flat-sequence {
              tunnel: [w1131] -> w1128
              tunnel: [w1130] -> w1127
              tunnel: [w1129] -> w1126
              tunnel: w1128 -> [w1139]
              tunnel: w1127 -> [w1138]
              tunnel: w1126 -> [w1137]
              tunnel: [w1138] -> w1125
              tunnel: [w1137] -> w1124
              tunnel: [w1136] -> w1123
              tunnel: w1125 -> [w1151]
              tunnel: w1124 -> [w1150]
              tunnel: w1123 -> [w1148]
              frame #0 {
                w1135 = TRUE ("可见")
                n734 = control-ref of="txtDrawingPrompt"() -> (w1134:refnum<vi>)
                n735 = control-ref of="ProgressNumerical"() -> (w1132:refnum<vi>)
                n736 = control-ref of="HorizontalProgressBar"() -> (w1133:refnum<vi>)
                n737 = property class="Slide (严格)"(reference=w1133, "Visible"=w1135) -> (reference out=w1130:refnum<vi>)  [unwired: 1 in, 1 out]
                n738 = property class="Str"(reference=w1132, "Visible"=w1135) -> (reference out=w1129:refnum<vi>)  [unwired: 1 in, 1 out]
                n739 = property class="Str"(reference=w1134, "Visible"=w1135) -> (reference out=w1131:refnum<vi>)  [unwired: 1 in, 1 out]
              }
              frame #1 {
                n740 = control-ref of="ArrySelectedSig"() -> (w1144:refnum<vi>)
                n741 = control-ref of="MainGraph"() -> (w1146:refnum<vi>)
                n742 = property class="XYGraph (严格)"(reference=w1146) -> ("Value"=w1145:cluster{"时间(s)":dbl[], "数据":dbl[]}[])  [unwired: 1 in, 2 out]
                n743 = property class="Arr (严格)"(reference=w1144) -> ("Value"=w1143:string[][])  [unwired: 1 in, 2 out]
                n744 = property class="Str"(reference=w1139, "Value"="通叔提示您：正在导出至EXCEL，请稍后..." ("key")) -> (reference out=w1136:refnum<vi>)  [unwired: 1 in, 1 out]
                n745 = Index Array(array=w1143, index (col)=1 ("禁用的索引 (列)")) -> (element=w1141:string[])  [unwired: 1 in]
                n746 = call "Export2Excel.vi"("进度数值"=w1137, "Slide输入"=w1138, "波形数组"=w1145, "信号名数组"=w1141) -> ()  [unwired: 8 in]
              }
              frame #2 {
                w1152 = FALSE ("可见")
                n747 = property class="Str"(reference=w1148, "Value"="" ("值")) -> (reference out=w1147:refnum<vi>)  [unwired: 1 in, 1 out]
                n748 = property class="Slide (严格)"(reference=w1151, "Visible"=w1152) -> ()  [unwired: 1 in, 2 out]
                n749 = property class="Str"(reference=w1150, "Visible"=w1152) -> ()  [unwired: 1 in, 2 out]
                n750 = property class="Str"(reference=w1147, "Visible"=w1152) -> ()  [unwired: 1 in, 2 out]
              }
            }
          }
          event Pane Size {
            n751 = event-data() -> ("OldBnds"=w1156:T26, "NewBnds"=w1157:T26)  [unwired: 1 in, 4 out]
            n752 = case shown="假" FALSE {
              tunnel: w1157 -> [_ _]
              tunnel: w1156 -> [_ _]
              tunnel: w1155 -> [w1169 w1180]
              tunnel: w1153 -> [_ w1181]
              frame False {
                n753 = control-ref of="boolExport2Excel"() -> (w1163:refnum<vi>)
                n754 = control-ref of="本VI"() -> (w1168:refnum<vi>)
                n755 = property class="VI"(reference=w1168) -> ("Front Panel.PanelBounds"=w1174:T26)  [unwired: 1 in, 2 out]
                n756 = Unbundle By Name(w1174) -> ("Right"=w1173:i16, "Left"=w1172:i16)
                n757 = property class="Bool"(reference=w1163) -> ("Top"=w1159:i32)  [unwired: 1 in, 2 out]
                n758 = Subtract(x=w1173, y=w1172) -> (x-y=w1171:i16)
                n759 = Divide(x=w1171, y=i16 9) -> (x/y=w1167:dbl)
                n760 = To Unsigned Long Integer(number=w1167) -> (unsigned 32bit integer=w1166:u32)
                n761 = property class="XYGraph (严格)"(reference=w1169, "LegWidth"=w1166) -> (reference out=w1165:refnum<vi>)  [unwired: 1 in, 1 out]
                n762 = property class="XYGraph (严格)"(reference=w1165) -> (reference out=w1160:refnum<vi>, "LegTop"=w1164:i32, "LegHt"=w1158:u32)  [unwired: 1 in, 1 out]
                n763 = Add(x=w1164, y=w1158) -> (x+y=w1162:u32)
                n764 = Greater?(x=w1162, y=w1159) -> (0:w1161:bool)
                n765 = case shown="真" w1161 {
                  tunnel: w1160 -> [_ w1179]
                  tunnel: w1159 -> [_ w1178]
                  tunnel: w1158 -> [_ w1177]
                  frame False {
                  }
                  frame True {
                    # "干涉了"
                    n766 = Subtract(x=w1178, y=w1177) -> (x-y=w1176:u32)
                    n767 = Decrement(x=w1176) -> (x-1=w1175:u32)
                    n768 = property class="XYGraph (严格)"(reference=w1179, "LegTop"=w1175) -> ()  [unwired: 1 in, 2 out]
                  }
                }
              }
              frame True {
                n769 = call "AdjustXYLegend.vi"("SelectedSigList"=w1181, "XYGraph输入"=w1180) -> ()  [unwired: 10 in]
              }
            }
          }
          event Value Change {
            n770 = event-data() -> ()  [unwired: 1 in, 6 out]
            n771 = flat-sequence {
              frame #0 {
                n772 = call "About.vi"() -> ()  [unwired: 11 in]
              }
              frame #1 {
                n773 = global read "GlobalVar.vi" "UserGroup"() -> (w1185:string)
                n774 = global read "GlobalVar.vi" "Language"() -> (w1187:u32)
                n775 = case shown="409, 默认" w1187 {
                  tunnel: [w1190 " [CAN协议与数据离线分析平台]-by 许晓通 QQ:19627152"] -> w1182
                  tunnel: [w1189 w1191] -> w1183
                  tunnel: w1185 -> [w1189 w1192]
                  frame 409, Default {
                    w1190 = " [CAN Offline Analysis Platform]-by Jay Sur E-mail:jaysur@foxmail.com"  # [CAN Offline Analysis Platform]-by Jay Sur E-mail:jaysur@foxmail.com
                  }
                  frame 804 {
                    n776 = case shown="\"SVIP\"" w1192 {
                      tunnel: ["普通用户" "VIP用户" "SVIP用户"] -> w1191
                      frame "假", Default {
                      }
                      frame "VIP" {
                      }
                      frame "SVIP" {
                      }
                    }
                  }
                }
                n777 = Concatenate Strings("X-CAN ", w1183, w1182) -> (w1186:string)
                n778 = control-ref of="本VI"() -> (w1188:refnum<vi>)
                n779 = property class="VI"(reference=w1188, "Front Panel.Title"=w1186) -> ()  [unwired: 1 in, 2 out]
              }
            }
          }
          event Menu Selection (User) {
            n780 = event-data() -> ("ItemTag"=w1197:string)  [unwired: 1 in, 6 out]
            n781 = case shown="\"MenuAbout\"" w1197 {
              frame "假", Default {
              }
              frame "openDBCedit" {
                n782 = call "openCANdb++.vi"() -> ()  [unwired: 12 in]
              }
              frame "ChkUpdate" {
                n783 = call <vilib>:"Application Directory.vi"() -> ("Application Directory"=w1202:path)
                n784 = Build Path(base path=w1202, name or relative path="updater.exe") -> (appended path=w1201:path)
                n785 = Path To String(path=w1201) -> (string=w1200:string)
                n786 = call <vilib>:"System Exec.vi"("wait until completion? (T)"=FALSE, "working directory"=w1202, "command line"=w1200) -> ("error out"=w1198:errorcluster)  [unwired: 5 in, 3 out]
                n787 = case shown="错误" w1198 {
                  frame No Error {
                  }
                  frame Error {
                    n788 = call "显示对话框信息6"() -> ()  [unwired: 10 in, 2 out]
                  }
                }
              }
              frame "MenuImportDBC" {
                n789 = call "文件对话框"("button label"="导入dbc", "pattern (all files)"="*.dbc" ("pattern label"), "pattern label"="dbc文件") -> ("selected path"=w1206:path)  [unwired: 9 in, 3 out]
                n790 = control-ref of="DBCpath"() -> (w1207:refnum<vi>)
                n791 = property class="Path"(reference=w1207, "Val(Sgnl)"=w1206) -> ()  [unwired: 1 in, 2 out]
              }
              frame "MenuImportCAN" {
                n792 = call "文件对话框2"("button label"="导入dbc", "pattern (all files)"=".can;*.csv;*.txt;*.asc" ("pattern label"), "pattern label"="CAN File") -> ("selected path"=w1212:path)  [unwired: 9 in, 3 out]
                n793 = control-ref of="CANpath"() -> (w1209:refnum<vi>)
                n794 = property class="Path"(reference=w1209, "Val(Sgnl)"=w1212) -> ()  [unwired: 1 in, 2 out]
              }
              frame "MenuCANjoiner" {
                n795 = call "CANjoiner.vi"() -> ()  [unwired: 12 in]
              }
              frame "MenuAbout" {
                n796 = call "About.vi"() -> ()  [unwired: 11 in]
              }
              frame "MenuDonate" {
                n797 = call "Donate.vi"() -> ()  [unwired: 12 in]
              }
            }
          }
          event Value Change {
            n798 = event-data() -> ()  [unwired: 1 in, 6 out]
            n799 = call "Donate.vi"() -> ()  [unwired: 12 in]
          }
          event "Language": Value Change {
            n800 = event-data() -> ()  [unwired: 1 in, 6 out]
            n801 = control-ref of="Language"() -> (w1215:refnum<vi>)
            n802 = control-ref of="本VI"() -> (w1214:refnum<vi>)
            n803 = call "UIinit_Main.vi"("VIref"=w1214, "Language"=w1215) -> ()  [unwired: 10 in]
          }
        }
      }
    }
  }
  n804 = control-ref of="SelectedSigValListArry"() -> (w9:refnum<vi>)
  n805 = control-ref of="XYGraphData"() -> (w8:refnum<vi>)
  n806 = control-ref of="MainGraph"() -> (w7:refnum<vi>)
  n807 = control-ref of="ArrySelectedSig"() -> (w10:refnum<vi>)
  n808 = control-ref of="XYTips"() -> (w12:refnum<vi>)
  n809 = node-c288() -> (w14:T22)  [unwired: 4 in]
  n810 = timed-loop {
    timing: w14 -> [_]
    timing-out: [_] -> w13
    tunnel: w12 -> [w1220]
    tunnel: w7 -> [w1219]
    tunnel: w10 -> [w1218]
    tunnel: w9 -> [w1217]
    tunnel: w8 -> [w1216]
    stop <- w1221 stop-if-true
    n811 = node-c288() -> ()  [unwired: 1 in, 1 out]
    n812 = event shown="[3] \"btnMultiDecAndExp\": 值改变" {
      selector: _ -> [_ _ _ _ _]
      dyn-events: _ -> [_ _ _ _ _]
      timeout: _ -> [_ _ _ _ _]
      tunnel: [_ TRUE _ _ _] -> w1221
      tunnel: w1220 -> [_ _ w1228 _ _]
      tunnel: w1219 -> [_ _ w1224 _ _]
      tunnel: w1218 -> [_ _ w1227 _ _]
      tunnel: w1217 -> [_ _ w1226 _ _]
      tunnel: w1216 -> [_ _ w1225 _ _]
      event Timeout {
        n813 = event-data() -> ()  [unwired: 1 in, 2 out]
      }
      event Panel Close {
        n814 = event-data() -> ()  [unwired: 1 in, 4 out]
      }
      event "MainGraph": Mouse Move {
        n815 = event-data() -> ("Coords"=w1229:T32)  [unwired: 1 in, 4 out]
        n816 = property on="isShowXY" class="Bool (严格)"() -> ("Value"=w1223:T5)  [unwired: 2 in, 2 out]
        n817 = case shown="真" w1223 {
          tunnel: w1229 -> [_ w1236]
          tunnel: w1228 -> [_ w1235]
          tunnel: w1227 -> [_ w1233]
          tunnel: w1226 -> [_ w1232]
          tunnel: w1225 -> [_ w1231]
          tunnel: w1224 -> [_ w1230]
          frame False {
          }
          frame True {
            n818 = invoke on="调用节点" class="XYGraph (严格)" method="GetPlotAtPos"(reference=w1230, "InputPt"=w1236) -> (reference out=w1237:refnum<vi>, "PlotNum"=w1234:i32)  [unwired: 3 in, 3 out]
            n819 = Greater?(x=w1234, y=-1) -> (0:w1238:bool)
            n820 = case shown="真" w1238 {
              tunnel: w1237 -> [_ w1254]
              tunnel: w1236 -> [_ w1252]
              tunnel: w1235 -> [w1240 w1253]
              tunnel: w1234 -> [_ w1244]
              tunnel: w1233 -> [_ w1251]
              tunnel: w1232 -> [_ w1248]
              tunnel: w1231 -> [_ w1246]
              tunnel: w1230 -> [_ w1242]
              frame False {
                n821 = property class="Str"(reference=w1240, "Visible"=FALSE ("可见")) -> ()  [unwired: 1 in, 2 out]
              }
              frame True {
                n822 = property class="Arr (严格)"(reference=w1248) -> ("Value"=w1247:string[][])  [unwired: 1 in, 2 out]
                n823 = property class="Arr (严格)"(reference=w1246) -> ("Value"=w1245:cluster{"时间(s)":dbl[], "数据":dbl[]}[])  [unwired: 1 in, 2 out]
                n824 = property class="Arr (严格)"(reference=w1251) -> ("Value"=w1250:string[][])  [unwired: 1 in, 2 out]
                n825 = Index Array(array=w1245, index=w1244) -> (element=w1243:cluster{"时间(s)":dbl[], "数据":dbl[]})
                n826 = Index Array(array=w1250, index (row)=w1244) -> (element=w1249:string[])  [unwired: 1 in]
                n827 = stacked-sequence {
                  seq-local: [_ w1268 _ _ _] -> [_ _ w1364 _ _]
                  seq-local: [_ w1266 _ _ _] -> [_ _ w1363 _ _]
                  seq-local: [_ w1267 _ _ _] -> [_ _ w1362 _ _]
                  tunnel: w1254 -> [w1259 w1280 _ w1374 _]
                  tunnel: w1253 -> [w1257 _ w1365 w1375 w1378]
                  tunnel: w1252 -> [w1256 w1281 _ _ _]
                  tunnel: w1244 -> [w1260 _ _ _ _]
                  tunnel: w1249 -> [_ w1277 _ _ _]
                  tunnel: w1247 -> [_ w1274 _ _ _]
                  tunnel: w1243 -> [_ w1262 _ _ _]
                  tunnel: w1242 -> [w1255 _ _ _ _]
                  frame #0 {
                    n828 = property on="属性节点" class="XYGraph (严格)"(reference=w1259, "Active Plot"=w1260) -> ()  [unwired: 1 in, 2 out]
                    n829 = call "Set_Tips_Position_XY.vi"("XYGraph输入"=w1255, "Offset"=u8 5, "Coords"=w1256, "TipsRef"=w1257) -> ()  [unwired: 8 in]
                  }
                  frame #1 {
                    n830 = property class="XYGraph (严格)"(reference=w1280) -> ("Plot.YScaleIdx"=w1279:u32)  [unwired: 1 in, 2 out]
                    n831 = property on="isShowYValue" class="Bool (严格)"() -> ("Value"=w1261:T5)  [unwired: 2 in, 2 out]
                    n832 = Index Array(array=w1274, index (col) #1=0 ("禁用的索引 (列)"), index (col) #2=2 ("禁用的索引 (行)"), index (col) #3=3 ("禁用的索引 (列)")) -> (element #1=w1271:string[], element #2=w1270:string[], element #3=w1263:string[])  [unwired: 3 in]
                    n833 = Index Array(array=w1277, index #1=15 ("禁用的索引 (列)"), index #2=0 ("索引")) -> (element #1=w1278:string, element #2=w1272:string)
                    n834 = invoke on="调用节点" class="XYGraph (严格)" method="Map Coords To XY"(reference=w1280, "Coords"=w1281, "Y Scale"=w1279) -> ("XY"=w1282:cluster{"X":dbl, "Y":dbl})  [unwired: 4 in, 6 out]
                    n835 = Unbundle By Name(w1282) -> ("X"=w1268:dbl, "Y"=w1269:dbl)
                    n836 = case shown="假" w1261 {
                      tunnel: w1278 -> [_ w1296]
                      tunnel: w1272 -> [_ w1295]
                      tunnel: w1271 -> [_ w1294]
                      tunnel: w1270 -> [_ w1293]
                      tunnel: w1269 -> [w1283 w1292]
                      tunnel: w1268 -> [_ w1291]
                      tunnel: ["" w1290] -> w1267
                      tunnel: [w1284 w1289] -> w1266
                      tunnel: w1263 -> [_ w1288]
                      tunnel: w1262 -> [_ w1287]
                      frame False {
                        n837 = Number To Fractional String(number=w1283, precision (6)=i16 3) -> (F-format string=w1284:string)  [unwired: 2 in]
                      }
                      frame True {
                        n838 = case shown="\"0\", 默认" w1296 {
                          tunnel: ["" w1308] -> w1290
                          tunnel: w1295 -> [_ w1306]
                          tunnel: w1294 -> [_ w1307]
                          tunnel: w1293 -> [_ w1305]
                          tunnel: w1288 -> [_ w1304]
                          tunnel: w1292 -> [w1298 _]
                          tunnel: w1291 -> [_ w1303]
                          tunnel: [w1297 w1302] -> w1289
                          tunnel: w1287 -> [_ w1301]
                          frame "0", Default {
                            n839 = Number To Fractional String(number=w1298, precision (6)=i16 3) -> (F-format string=w1297:string)  [unwired: 2 in]
                          }
                          frame "1" {
                            n840 = stacked-sequence {
                              seq-local: [_ w1319 _] -> [_ _ w1350]
                              seq-local: [_ w1318 _] -> [_ _ w1358]
                              seq-local: [_ w1316 _] -> [_ _ w1352]
                              seq-local: [w1309 _ _] -> [_ _ w1349]
                              tunnel: [_ _ w1355] -> w1308
                              tunnel: w1307 -> [_ w1324 _]
                              tunnel: w1306 -> [_ w1321 _]
                              tunnel: w1305 -> [_ w1323 _]
                              tunnel: w1304 -> [_ w1322 _]
                              tunnel: w1303 -> [w1313 _ _]
                              tunnel: [_ _ w1351] -> w1302
                              tunnel: w1301 -> [w1315 _ _]
                              frame #0 {
                                n841 = Unbundle(w1315) -> ("时间(s)"=w1314:dbl[], "数据"=w1310:dbl[])
                                n842 = Threshold 1D Array(2:w1313, 3:w1314) -> (0:w1312:dbl)  [unwired: 1 in]
                                n843 = Round Toward -Infinity(1:w1312) -> (0:w1311:dbl)
                                n844 = Index Array(array=w1310, index=w1311) -> (element=w1309:dbl)
                              }
                              frame #1 {
                                w1317 = string[] []
                                n845 = for {
                                tunnel: w1324 -> [w1334] mode=indexing
                                tunnel: w1323 -> [w1333] mode=indexing
                                tunnel: w1322 -> [w1329] mode=indexing
                                tunnel: w1321 -> [w1335]
                                shift-right: [w1332] -> w1319
                                shift-left: dbl[] [] -> [w1331]
                                shift-right: [w1328] -> w1318
                                shift-left: w1317 -> [w1327]
                                shift-right: [w1326] -> w1316
                                shift-left: w1317 -> [w1325]
                                n846 = Equal?(x=w1335, y=w1334) -> (x = y?=w1330:bool)
                                n847 = case shown="真" w1330 {
                                tunnel: w1333 -> [_ w1341]
                                tunnel: [w1338 w1346] -> w1332
                                tunnel: w1331 -> [w1338 w1345]
                                tunnel: w1329 -> [_ w1344]
                                tunnel: [w1337 w1343] -> w1328
                                tunnel: w1327 -> [w1337 w1342]
                                tunnel: [w1336 w1340] -> w1326
                                tunnel: w1325 -> [w1336 w1339]
                                frame False {
                                }
                                frame True {
                                n848 = Fract/Exp String To Number(string=w1341) -> (number=w1347:dbl)  [unwired: 3 in, 1 out]
                                n849 = Build Array (concatenate)(w1345, w1347) -> (w1346:dbl[])
                                n850 = Build Array (concatenate)(w1339, w1341) -> (w1340:string[])
                                n851 = Build Array (concatenate)(w1342, w1344) -> (w1343:string[])
                                }
                                }
                                }
                              }
                              frame #2 {
                                n852 = Search 1D Array(1D array=w1350, element=w1349) -> (index of element=w1348:i32)  [unwired: 1 in]
                                n853 = Index Array(array=w1358, index=w1348) -> (element=w1354:string)
                                n854 = Concatenate Strings("(" ("string"), w1354, ")" ("字符串")) -> (w1356:string)
                                n855 = Empty String/Path?(string/path=w1354) -> (empty?=w1353:bool)
                                n856 = case shown="真" w1353 {
                                tunnel: w1356 -> [w1360 _]
                                tunnel: [w1360 ""] -> w1355
                                frame False {
                                }
                                frame True {
                                }
                                }
                                n857 = Index Array(array=w1352, index=w1348) -> (element=w1351:string)
                              }
                            }
                          }
                        }
                      }
                    }
                  }
                  frame #2 {
                    n858 = Number To Fractional String(number=w1364, precision (6)=i16 3 ("精度(6)")) -> (F-format string=w1368:string)  [unwired: 2 in]
                    n859 = Concatenate Strings("X : " ("string"), w1368) -> (w1372:string)
                    n860 = Concatenate Strings("Y : " ("string"), w1363) -> (w1369:string)
                    n861 = Concatenate Strings(w1372, "\r", w1369, w1362) -> (w1367:string)
                    n862 = property class="Str"(reference=w1365, "Value"=w1367) -> ()  [unwired: 1 in, 2 out]
                  }
                  frame #3 {
                    n863 = property on="属性节点" class="XYGraph (严格)"(reference=w1374) -> ("Plot.Plot Color"=w1376:u32)  [unwired: 1 in, 2 out]
                    n864 = property on="属性节点" class="Str"(reference=w1375, "Text.TextColor"=w1376) -> ()  [unwired: 1 in, 2 out]
                  }
                  frame #4 {
                    n865 = property class="Str"(reference=w1378, "Visible"=TRUE ("可见")) -> ()  [unwired: 1 in, 2 out]
                  }
                }
              }
            }
          }
        }
      }
      event "btnMultiDecAndExp": Value Change {
        n866 = event-data() -> ()  [unwired: 1 in, 6 out]
        n867 = local read "NumSelected"() -> (w1383:i32)
        n868 = local read "DBC_loaded"() -> (w1380:bool)
        n869 = control-ref of="txtDrawingPrompt"() -> (w1379:refnum<vi>)
        n870 = Greater Than 0?(x=w1383) -> (x > 0?=w1382:bool)
        n871 = And(x=w1380, y=w1382) -> (x .and. y?=w1381:bool)
        n872 = case shown="真" w1381 {
          tunnel: w1380 -> [w1384 _]
          tunnel: w1379 -> [_ w1385]
          frame False {
            n873 = case shown="假" w1384 {
              frame False {
                n874 = call "显示对话框信息2"() -> ()  [unwired: 10 in, 2 out]
              }
              frame True {
                n875 = call "显示对话框信息13"() -> ()  [unwired: 10 in, 2 out]
              }
            }
          }
          frame True {
            n876 = stacked-sequence {
              seq-local: [w1389 _ _] -> [_ w1425 w1494]
              seq-local: [w1393 _ _] -> [_ w1426 _]
              seq-local: [w1392 _ _] -> [_ w1424 _]
              seq-local: [_ w1423 _] -> [_ _ w1499]
              seq-local: [_ w1422 _] -> [_ _ w1492]
              tunnel: w1385 -> [w1391 w1421 w1498]
              frame #0 {
                n877 = global read "GlobalVariables.vi" "可识别数据类型"() -> (w1395:string)
                n878 = call "文件对话框5"("pattern (all files)"=w1395, "pattern label"="CAN文件") -> ("selected paths"=w1389:path[], "error out"=w1409:errorcluster)  [unwired: 10 in, 2 out]
                n879 = Array Size(array=w1389) -> (size(s)=w1387:i32)
                n880 = Format Into String(format string="准备解析%d个文件。" ("格式字符串"), w1387) -> (resulting string=w1388:string)  [unwired: 2 in, 1 out]
                n881 = property class="Str"(reference=w1391, "Visible"=TRUE ("可见"), "Value"=w1388) -> ()  [unwired: 1 in, 2 out]
                n882 = Concatenate Strings("解析的文件列表：" ("字符串"), "\r\n") -> (w1398:string)
                n883 = call <vilib>:"New Report.vi"("window state (normal)"=T38."minimized", "report type"=T39."Excel", "error in (no error)"=w1409) -> ("report out"=w1403:refnum<class "NI_report.lvclass">, "error out"=w1402:errorcluster)  [unwired: 11 in]
                n884 = for {
                  tunnel: w1389 -> [w1420] mode=indexing
                  shift-right: [w1415] -> w1407
                  shift-left: w1398 -> [w1416]
                  i -> [w1414]
                  n885 = Strip Path(path=w1420) -> (name=w1418:string)  [unwired: 1 out]
                  n886 = Increment(x=w1414) -> (x+1=w1413:i32)
                  n887 = Format Into String(format string="文件%d：" ("字符串"), w1413) -> (resulting string=w1411:string)  [unwired: 2 in, 1 out]
                  n888 = Concatenate Strings(w1416, w1411, "\t", w1418, "\r\n") -> (w1415:string)
                }
                n889 = call <vilib>:"Excel Rename Worksheet.vi"("report in"=w1403, "worksheet name (\"\")"="文件列表" ("worksheet name (\"\")"), "error in (no error)"=w1402) -> ("report out"=w1399:refnum<class "NI_report.lvclass">, "error out"=w1400:errorcluster)  [unwired: 11 in]
                n890 = Spreadsheet String To Array(format string="%s" ("格式字符串"), spreadsheet string=w1407, array type (2D Dbl)=string[][] []) -> (array=w1404:string[][])  [unwired: 1 in]
                n891 = call-poly <vilib>:"Append Table to Report.vi"("report in"=w1399, "text data"=w1404, "error in (no error)"=w1400) -> ("report out"=w1393:refnum<class "NI_report.lvclass">, "error out"=w1392:errorcluster)  [unwired: 9 in, 2 out]
              }
              frame #1 {
                n892 = for {
                  shift-right: [w1431] -> w1423
                  shift-left: w1426 -> [w1440]
                  shift-right: [w1432] -> w1422
                  shift-left: w1424 -> [w1438]
                  tunnel: w1425 -> [w1439] mode=indexing
                  tunnel: w1421 -> [w1430]
                  i -> [w1428]
                  n893 = call <vilib>:"Get File Extension.vi"("error in (no error)"=w1438, "file"=w1439) -> ("error out"=w1449:errorcluster, "dup file"=w1435:path)  [unwired: 5 in, 3 out]
                  n894 = call <vilib>:"Excel Add Worksheet.vi"("report in"=w1440, "error in (no error)"=w1449) -> ("report out"=w1445:refnum<class "NI_report.lvclass">, "error out"=w1446:errorcluster)  [unwired: 12 in]
                  n895 = Format Into String(format string="正在解析第%d个" ("格式字符串"), w1428) -> (resulting string=w1429:string)  [unwired: 2 in, 1 out]
                  n896 = Increment(x=w1428) -> (x+1=w1441:i32)
                  n897 = control-ref of="ProgressNumerical"() -> (w1434:refnum<vi>)
                  n898 = control-ref of="HorizontalProgressBar"() -> (w1433:refnum<vi>)
                  n899 = call <vilib>:"Excel Get Worksheet.vi"("report in"=w1445, "worksheet index (0)"=w1441, "error in (no error)"=w1446) -> ("report out"=w1448:refnum<class "NI_report.lvclass">, "error out"=w1447:errorcluster)  [unwired: 11 in]
                  n900 = property class="Str"(reference=w1430, "Value"=w1429) -> ()  [unwired: 1 in, 2 out]
                  n901 = Format Into String(format string="%d" ("格式字符串"), initial string="文件" ("初始字符串"), w1441) -> (resulting string=w1442:string)  [unwired: 1 in, 1 out]
                  n902 = call <vilib>:"Excel Rename Worksheet.vi"("report in"=w1448, "worksheet name (\"\")"=w1442, "error in (no error)"=w1447) -> ("report out"=w1437:refnum<class "NI_report.lvclass">, "error out"=w1436:errorcluster)  [unwired: 11 in]
                  n903 = stacked-sequence {
                    seq-local: [_ _ _ _ _ w1466 _ _] -> [_ _ _ _ _ _ w1473 _]
                    tunnel: w1437 -> [_ _ _ _ _ _ w1475 _]
                    tunnel: w1436 -> [_ _ _ _ _ _ w1474 _]
                    tunnel: w1435 -> [w1450 _ _ _ _ _ _ _]
                    tunnel: w1434 -> [_ _ _ _ w1460 w1464 _ w1476]
                    tunnel: w1433 -> [_ _ _ _ w1459 w1465 _ w1477]
                    tunnel: [_ _ _ _ _ _ w1472 _] -> w1432
                    tunnel: [_ _ _ _ _ _ w1471 _] -> w1431
                    frame #0 {
                      n904 = control-ref of="CANpath"() -> (w1452:refnum<vi>)
                      n905 = local write "Data_loaded"(FALSE ("Data_loaded")) -> ()
                      n906 = property class="Path"(reference=w1452, "Val(Sgnl)"=w1450) -> ()  [unwired: 1 in, 2 out]
                    }
                    frame #1 {
                      n907 = while {
                        stop <- w1453 stop-if-true
                        n908 = local read "Data_loaded"() -> (w1453:bool)
                      }
                    }
                    frame #2 {
                      n909 = local read "boolDrawGraph"() -> (w1457:bool)
                      n910 = local write "MainGrapgDraw_finished"(FALSE ("MainGrapgDraw_finished")) -> ()
                      n911 = Not(x=w1457) -> (.not. x?=w1455:bool)
                      n912 = control-ref of="boolDrawGraph"() -> (w1456:refnum<vi>)
                      n913 = property class="Bool (严格)"(reference=w1456, "Val(Sgnl)"=w1455) -> ()  [unwired: 1 in, 2 out]
                    }
                    frame #3 {
                      n914 = while {
                        stop <- w1458 stop-if-true
                        n915 = local read "MainGrapgDraw_finished"() -> (w1458:bool)
                      }
                    }
                    frame #4 {
                      w1461 = TRUE ("可见")
                      n916 = property class="Slide (严格)"(reference=w1459, "Visible"=w1461) -> ()  [unwired: 1 in, 2 out]
                      n917 = property class="Str"(reference=w1460, "Visible"=w1461) -> ()  [unwired: 1 in, 2 out]
                    }
                    frame #5 {
                      n918 = control-ref of="MainGraph"() -> (w1463:refnum<vi>)
                      n919 = control-ref of="ArrySelectedSig"() -> (w1462:refnum<vi>)
                      n920 = property class="XYGraph (严格)"(reference=w1463) -> ("Value"=w1467:cluster{"时间(s)":dbl[], "数据":dbl[]}[])  [unwired: 1 in, 2 out]
                      n921 = property class="Arr (严格)"(reference=w1462) -> ("Value"=w1470:string[][])  [unwired: 1 in, 2 out]
                      n922 = Index Array(array=w1470, index (col)=1 ("禁用的索引 (列)")) -> (element=w1468:string[])  [unwired: 1 in]
                      n923 = call "Export2SheetString.vi"("波形数组"=w1467, "信号名数组"=w1468, "进度数值"=w1464, "Slide输入"=w1465) -> ("SheetSpread"=w1466:string[][])  [unwired: 7 in]
                    }
                    frame #6 {
                      n924 = call-poly <vilib>:"Append Table to Report.vi"("report in"=w1475, "text data"=w1473, "error in (no error)"=w1474) -> ("report out"=w1471:refnum<class "NI_report.lvclass">, "error out"=w1472:errorcluster)  [unwired: 9 in, 2 out]
                    }
                    frame #7 {
                      w1478 = FALSE ("可见")
                      n925 = property class="Slide (严格)"(reference=w1477, "Visible"=w1478) -> ()  [unwired: 1 in, 2 out]
                      n926 = property class="Str"(reference=w1476, "Visible"=w1478) -> ()  [unwired: 1 in, 2 out]
                    }
                  }
                }
              }
              frame #2 {
                n927 = Index Array(array=w1494, index=0 ("索引")) -> (element=w1490:path)
                n928 = Array Size(array=w1494) -> (size(s)=w1486:i32)
                n929 = Strip Path(path=w1490) -> (stripped path=w1489:path)  [unwired: 1 out]
                n930 = Get Date/Time In Seconds() -> (seconds since 1Jan1904=w1488:timestamp)
                n931 = property class="Str"(reference=w1498, "Value"="解析并导出完成。" ("值")) -> (reference out=w1496:refnum<vi>)  [unwired: 1 in, 1 out]
                n932 = Format Date/Time String(time format string (%c)="%Y%m%d%H%M" ("时间格式字符串(%c)"), seconds (now)=w1488) -> (date/time string=w1484:string)  [unwired: 1 in]
                n933 = Format Into String(format string="多文件解析_%d文件_%s.xls" ("格式字符串"), w1486, w1484) -> (resulting string=w1483:string)  [unwired: 2 in, 1 out]
                n934 = Build Path(base path=w1489, name or relative path=w1483) -> (appended path=w1491:path)
                n935 = property class="Str"(reference=w1496, "Visible"=FALSE ("可见")) -> ()  [unwired: 1 in, 2 out]
                n936 = call-dynamic "Save Report to File.vi"("report in"=w1499, "report file path"=w1491, "error in (no error)"=w1492) -> ("report out"=w1482:refnum<class "NI_report.lvclass">, "error out"=w1480:errorcluster)  [unwired: 11 in]
                n937 = call-dynamic "Dispose Report.vi"("report in"=w1482, "save changes? (F)"=TRUE, "error in (no error)"=w1480) -> ("error out"=w1479:errorcluster)  [unwired: 12 in]
                n938 = Path To String(path=w1491) -> (string=w1501:string)
                n939 = Concatenate Strings("cmd /c\"" ("字符串"), w1501, "\"" ("字符串")) -> (w1500:string)
                n940 = call <vilib>:"System Exec.vi"("run minimized? (F)"=TRUE, "error in (no error)"=w1479, "command line"=w1500) -> ()  [unwired: 5 in, 4 out]
              }
            }
          }
        }
      }
      event "MainGraph": Plot Attribute Change {
        n941 = event-data() -> ("CtlRef"=w1505:refnum<vi>, "OldAttrib"=w1510:T40, "NewAttrib"=w1506:T40)  [unwired: 1 in, 5 out]
        n942 = Unbundle By Name(w1510) -> ("Color"=w1509:u32)
        n943 = Unbundle By Name(w1506) -> ("Color"=w1508:u32)
        n944 = Not Equal?(x=w1509, y=w1508) -> (x != y?=w1507:bool)
        n945 = case shown="真" w1507 {
          tunnel: w1506 -> [_ w1513]
          tunnel: w1505 -> [_ w1514]
          frame False {
          }
          frame True {
            n946 = Unbundle By Name(w1513) -> ("YScaleIdx"=w1512:u32, "Color"=w1511:u32)
            n947 = property class="XYGraph (严格)"(reference=w1514, "ActYScl"=w1512, "YScale.NameLbl.TextColor"=w1511, "YScale.Text Color"=w1511, "YScale.TickColor"=w1511, "YScale.MinorTickColor"=w1511) -> ()  [unwired: 1 in, 2 out]
          }
        }
      }
    }
    n948 = node-c288() -> ()  [unwired: 1 in, 1 out]
  }
  n949 = node-c288(w20) -> ()  [unwired: 1 out]
  n950 = node-c288(w13) -> ()  [unwired: 1 out]
